vi "Main.vi"() -> ()   [LabVIEW 2017, in "CL_G3_BuilderApplicationLayer.lvlib"]
uses:
  CL_G3_BuilderApplicationLayer.lvlib
  TypeDefs/Organizational Types View.ctl
  TypeDefs/Email Behavior.ctl
  Message Queue/Message Cluster.ctl
  Build Analyzer/Build Analyzer.lvclass
  TypeDefs/Application Model Build States.ctl
  Exports/Exports/Export.lvclass
  <userlib>/_Cirrus Logic/LabVIEW SCC API/Source/Abstract SCC/Abstract SCC API.lvclass
  Components/Component.lvclass
  Build Analyzer/Build Analyzer.lvclass/Build Analyzer.ctl
  Exports/Exports/Export.lvclass/Export.ctl
  Components/Component.lvclass/Component.ctl
  Commit Behavior/Commit/Commit.lvclass
  Commit Behavior/Commit/Commit.lvclass/Commit.ctl
  Build Analyzer/Accessors/Read Component Product Name -_ Unique Name.vi
  Build Analyzer/Accessors/Read Product Name - Unique Name.vi
  Exports/Exports/Accessors/Read Product Name.vi
  Exports/Exports/Accessors/Read Built Version.vi
  Exports/Exports/Accessors/Read Owning Component's Product Name.vi
  Components/Accessors/Read Component Operations Errors.vi
  Exports/Exports/Accessors/Read Commit behavior.vi
  Exports/Exports/Accessors/Read Component Root path.vi
  Exports/Exports/Accessors/Write Export Operation Errors.vi
  Exports/Exports/Accessors/Read Component Export Dir.vi
  Exports/Exports/Accessors/Read Export Artifacts for SCC.vi
  Exports/Exports/Accessors/Read unique Name.vi
  Commit Behavior/Commit/Accessors/Read Commit Operation Errors.vi
  Message Queue/Enqueue Message (Single).vi
  Message Queue/Enqueue Message (Array).vi
  <vilib>/smtpClient/Set Message Text.vi
  <vilib>/LVH/i3 JSON/JSON Parsing/Get Object Parameter Files/Get Object Parameter - Object.vi
  <vilib>/LVH/i3 JSON/JSON Parsing/Get Object Parameter Files/Get Object Parameter - Numeric.vi
  <vilib>/LVH/i3 JSON/JSON Parsing/Get Object Parameter Files/Get Object Parameter - Array.vi
  <vilib>/LVH/i3 JSON/JSON Parsing/Get Array Value at Index Files/Get Array Value at Index - String.vi
  <vilib>/LVH/i3 JSON/JSON Parsing/Get Object Parameter Files/Get Object Parameter - String.vi
  <userlib>/_OpenG.lib/array/array.llb/Filter 1D Array (String)__ogtk.vi
  <vilib>/ErrorRing/Error Ring.xnode
  Message Queue/Message Queue.lvlib
  <vilib>/smtpClient/LabVIEWSMTPClient.lvlib
  CL_G3_VIComponentBuilder.lvlib
  <vilib>/Utility/config.llb/NI_LVConfig.lvlib
  <vilib>/LVH/i3 JSON/i3-json.lvlib
panel:
  in  "Sender's Email Address":string
  in  "Outgoing Mail Server":string
  in  "Email Behavior":T1
  in  "Email Address":string[](array[string])
  in  "Component \\ Export View":T2=enum."Component View"
  in  "Auto Submit Behavior":T3(ring)=enum."No Auto Submit"
  in  "Sync Action":enum16{"No Sync", "Sync", "Force Sync"}(ring)=enum."Force Sync"
  out "error out":errorcluster
  in  "Shutdown":bool
  in  "Back":bool
  in  "Status":string="Analysis Complete. Select componets to build"
  in  "Next Button":bool
  in  "Build Phase":T4(tab)
  in  "Select all":bool
  in  "Select None":bool
  in  "Components to build":u16[](array[ring]) items=["Component Builder", "Component Template NIPKG VIP", "Custom Install Step Launcher", "LabVIEW Atlassian API", "LabVIEW Auto Documentation", "LabVIEW Container", "LabVIEW SCC API", "NI Package Manager API", "NI Package Manager Build Spec Utils"]
  in  "Build Type":T5(ring)
  in  "Exports":i32(listbox)=-1
  in  "Abort":bool
  in  "Failed Builds":i32(listbox)=-2
  in  "Successful Builds":i32(listbox)=-2
  in  "Submission Status":i32(listbox)
  # "Email Options"
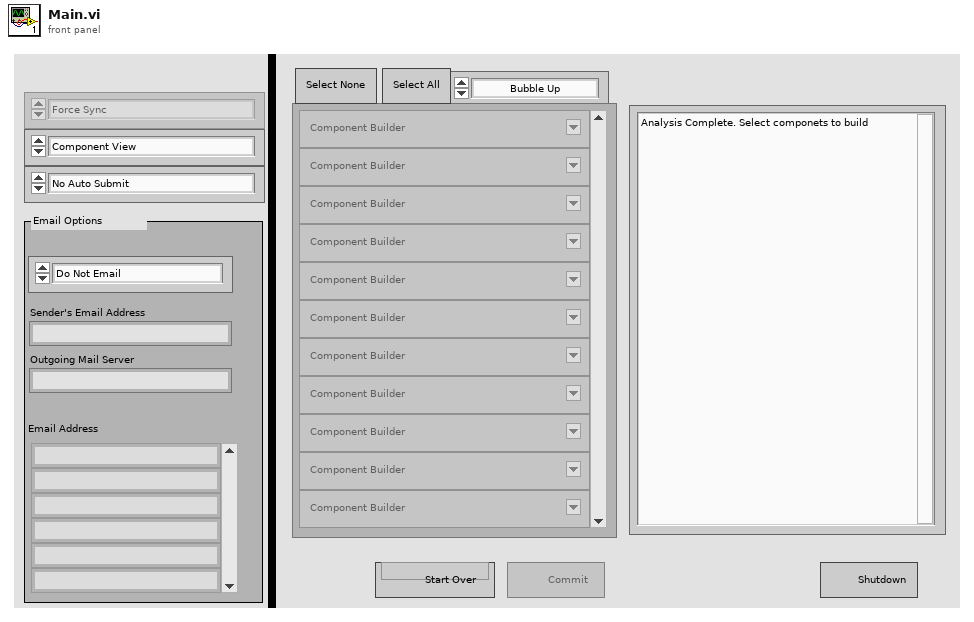
[diagram p1: front panel]
types:
  T1 = typedef "CL_G3_BuilderApplicationLayer.lvlib/Email Behavior.ctl" = enum16{"Do Not Email", "Email On Any Failure", "Email On All Successfully Built", "Email On Success OR Failure"}
  T2 = typedef "CL_G3_BuilderApplicationLayer.lvlib/Organizational Types View.ctl" = enum16{"Export View", "Component View"}
  T3 = enum16{"Auto Submit All Built Exports", "No Auto Submit"}
  T4 = enum32{"Configure Build", "Build Status", "Build Results", "Results"}
  T5 = enum16{"Bubble Up", "Build Dependencies", "Build Selected Only"}
  T6 = cluster{"This VI":refnum<vi>, "Build Analyzer":refnum<class "Build Analyzer.lvclass">, "Build Type":enum16{"Bubble Up", "Build Dependencies", "Build Selected Only"}, "Buildable Components":string[], "Components to Build":u16[], "Build Results":refnum<class "Export.lvclass">[], "Build Groups Folder":path, "View Type":T2, "Export Build Order":refnum<class "Export.lvclass">[], "Build Marker":u32, "Control References":cluster{"Auto Submit Behavior":refnum<vi>, "Email Address":refnum<vi>, "Outgoing Mail Server":refnum<vi>, "Sender's Email Address":refnum<vi>, "Sync Action":refnum<vi>, "Component \\ Export View Reference":refnum<vi>, "Email Behavior Reference":refnum<vi>, "Successful Builds":refnum<vi>, "Failed Builds":refnum<vi>, "Submission Status":refnum<vi>, "Shutdown":refnum<vi>, "Abort":refnum<vi>, "Front Panel":refnum<vi>, "Build Type":refnum<vi>, "Back":refnum<vi>, "Next":refnum<vi>, "Clear":refnum<vi>, "Select All":refnum<vi>, "Components to Build":refnum<vi>}}
  T7 = cluster{"SCC Session":refnum<class "Abstract SCC API.lvclass">, "Build Analyzer":refnum<class "Build Analyzer.lvclass">, "Ordered Exports":refnum<class "Export.lvclass">[], "Build Marker":u32, "Build Groups Folder":path, "Components":refnum<class "Component.lvclass">[], "Sync Action":enum16{"No Sync", "Sync", "Force Sync"}, "Build Options i3JSON Tree":variant, "Broadcast Server Id":refnum<k5>, "Failed Submissions":refnum<class "Export.lvclass">[], "All Attempted Submissions":refnum<class "Export.lvclass">[], "Successful Submissions":refnum<class "Export.lvclass">[], "SCC Synchronized Paths":variant, "Snapshot Depot Directories":string[]}
  T8 = typedef "CL_G3_BuilderApplicationLayer.lvlib/Application Model Build States.ctl" = enum32{"Configure Build", "Build Pre Check", "Build Status", "Build Results", "Finished"}
  T9 = cluster{"Dynamic Event":refnum<user-event>, "Build Analyzer":refnum<class "Build Analyzer.lvclass">, "Current Phase":T8, "Email Behavior":T1, "Export Build Order":refnum<class "Export.lvclass">[]}
  T10 = typedef "CL_G3_BuilderApplicationLayer.lvlib/Message Queue.lvlib/Message Cluster.ctl" = cluster{"Message":string, "Message Data":variant}
  T11 = typedef "CL_G3_BuilderApplicationLayer.lvlib/Message Queue.lvlib/All Message Queues.ctl" = cluster{"UI":refnum<queue>, "Application Model":refnum<queue>, "UI manager":refnum<queue>, "Build Engine":refnum<queue>}
  T12 = enum8{"Enabled", "Disabled", "Disabled and Grayed Out"}
  T13 = cluster{"Ordered Exports":refnum<class "Export.lvclass">[], "Build Groups Folder":path}
  T14 = typedef "LabVIEWSMTPClient.lvlib/SmtpClientHandle.ctl" = refnum<k1>
  T15 = cluster{"Ordered Exports":refnum<class "Export.lvclass">[], "Build Marker":u32, "Build Groups Folder":path, "Build Engine Queue":refnum<queue>, "error out":errorcluster}
  T16 = cluster{"Export Path":path, "Export Files":string[]}
  T17 = typedef "NI_LVConfig.lvlib/Config Data RefNum.ctl" = refnum<k1>
  T18 = cluster{"SCC Session":refnum<class "Abstract SCC API.lvclass">, "Failed Submissions":refnum<class "Export.lvclass">[], "All Exports":refnum<class "Export.lvclass">[], "Exports W\\O Errors":refnum<class "Export.lvclass">[], "Ordered Expors":refnum<class "Export.lvclass">[]}
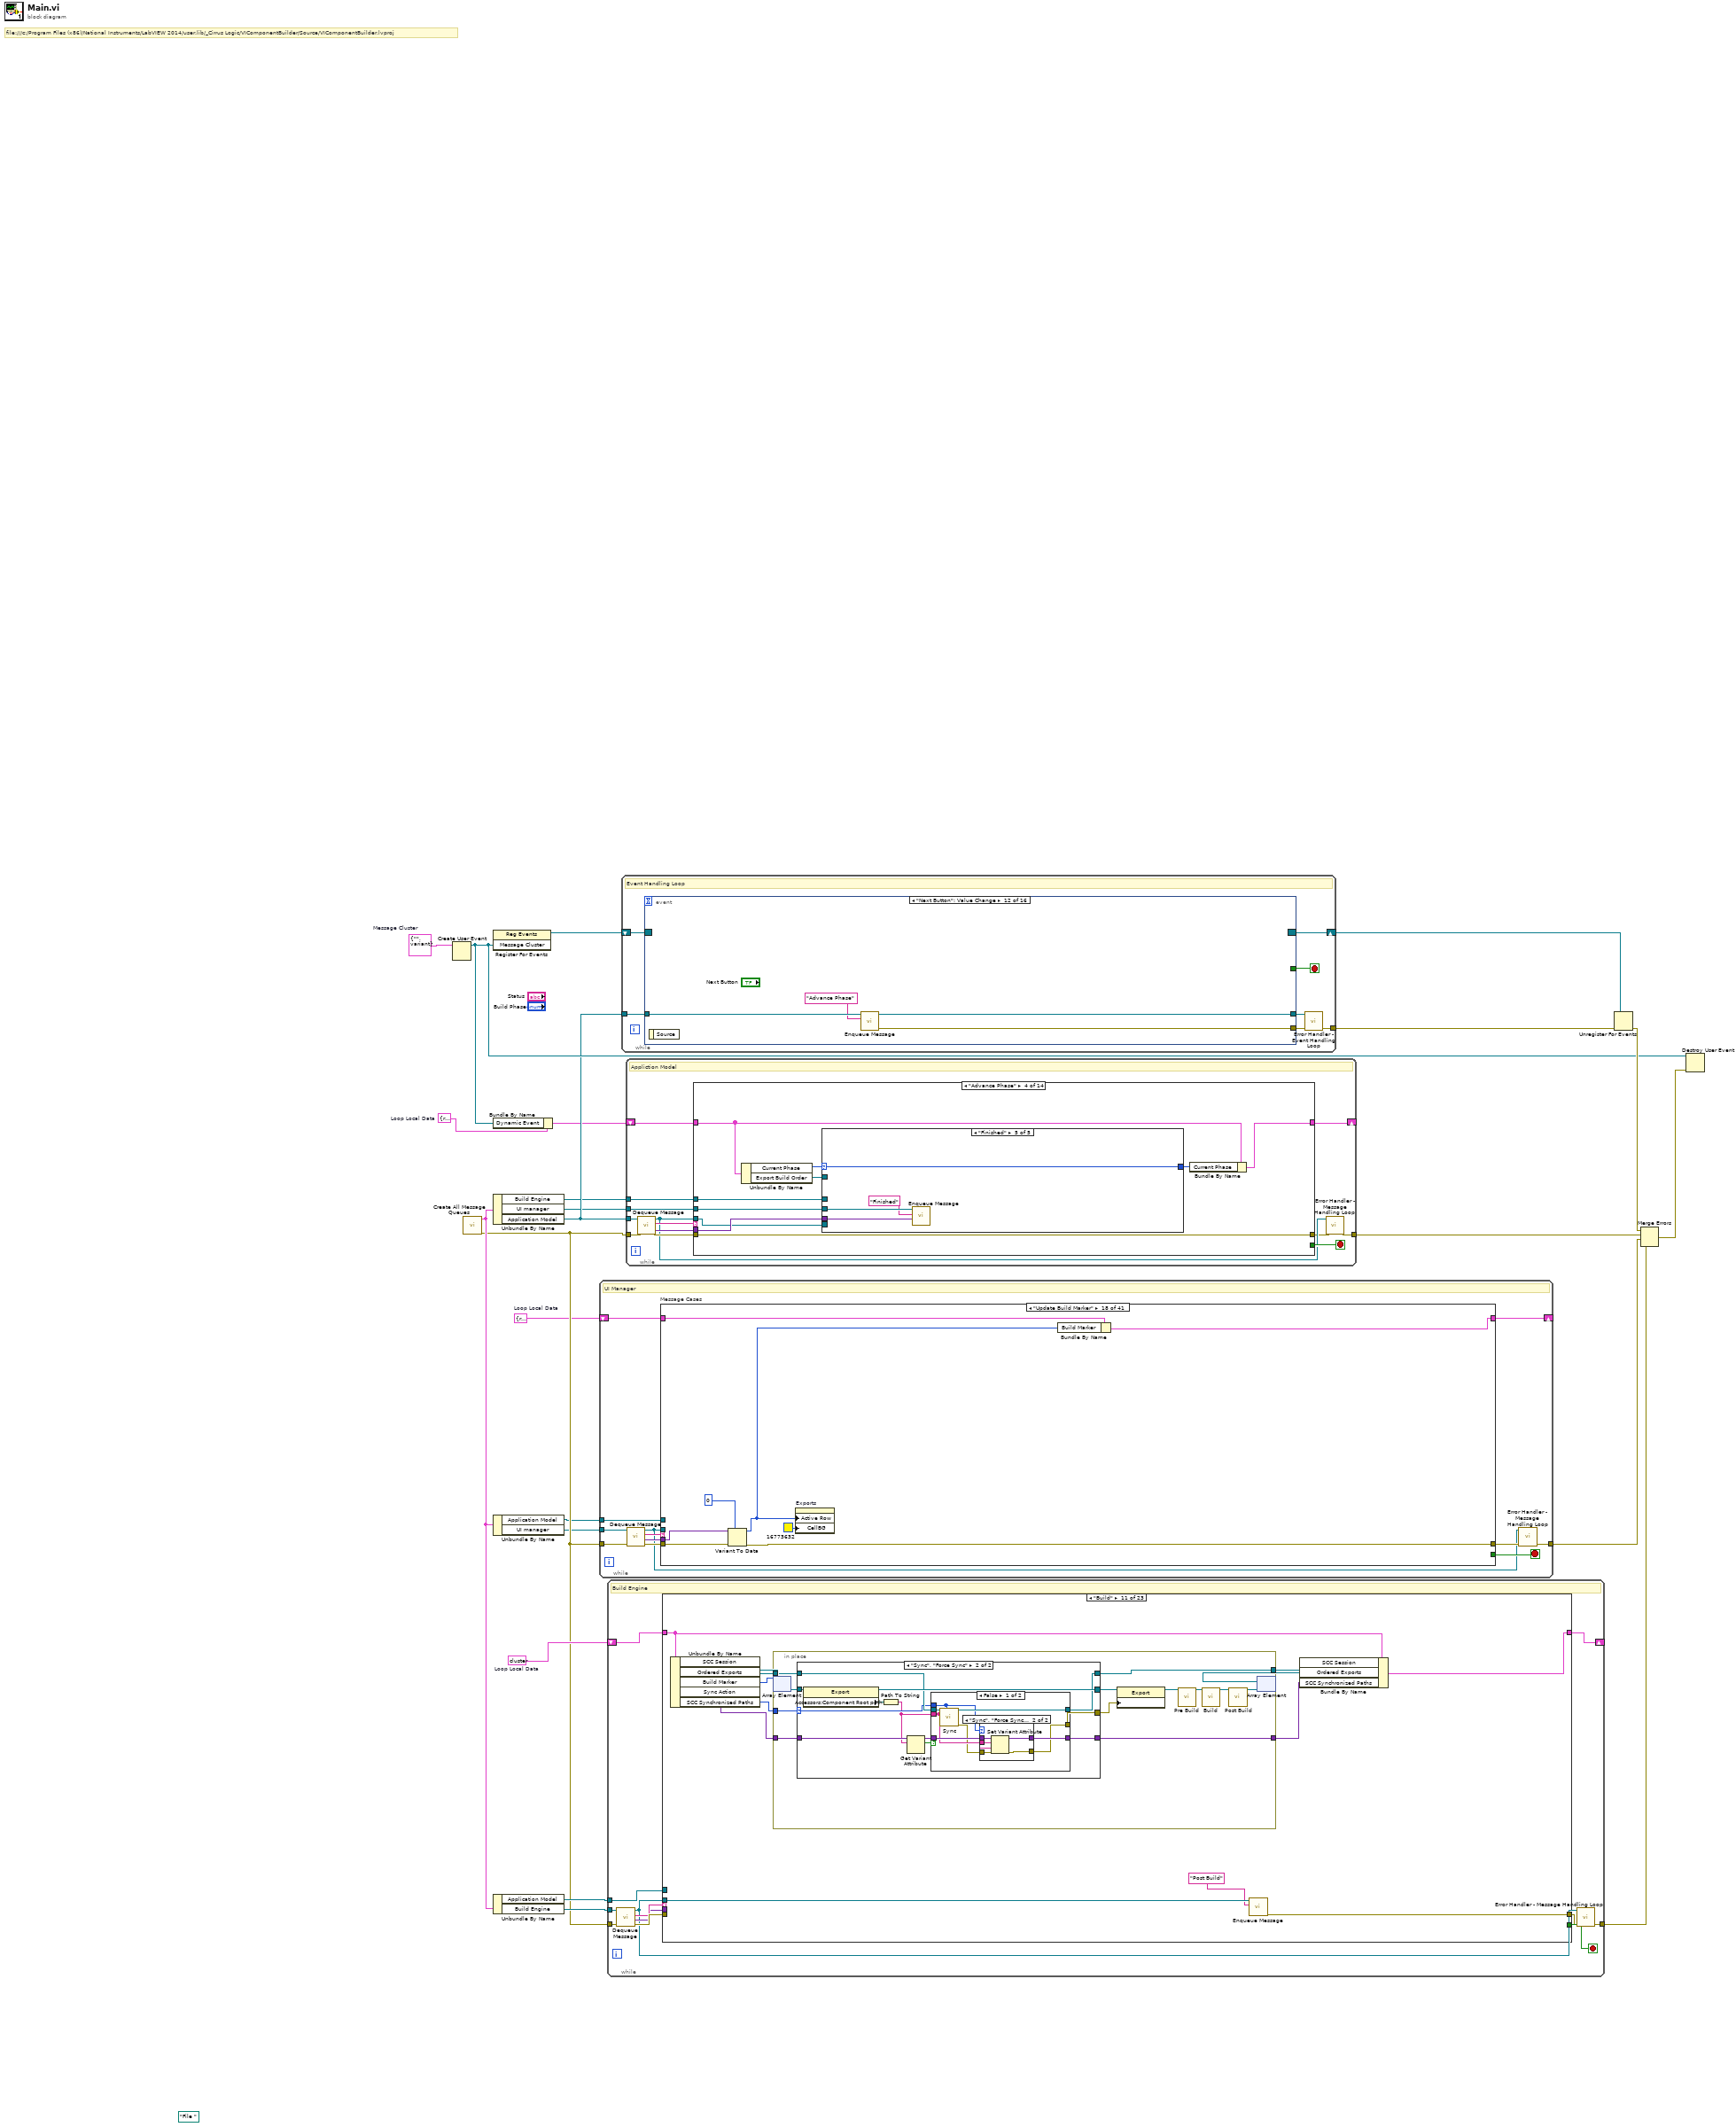
[diagram p0: block diagram]
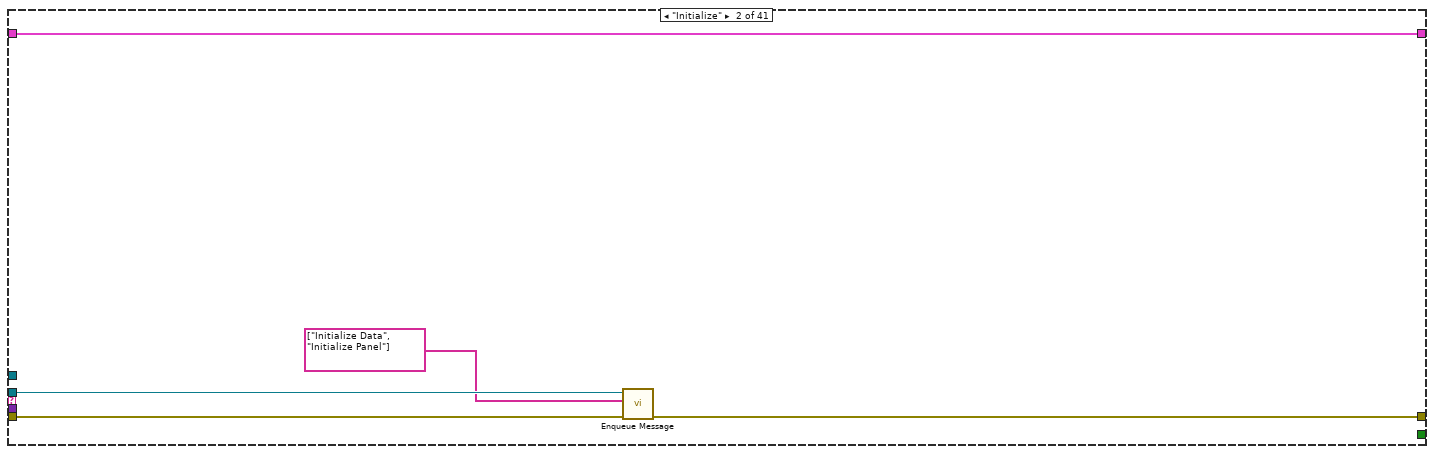
[diagram p3: hidden frame]
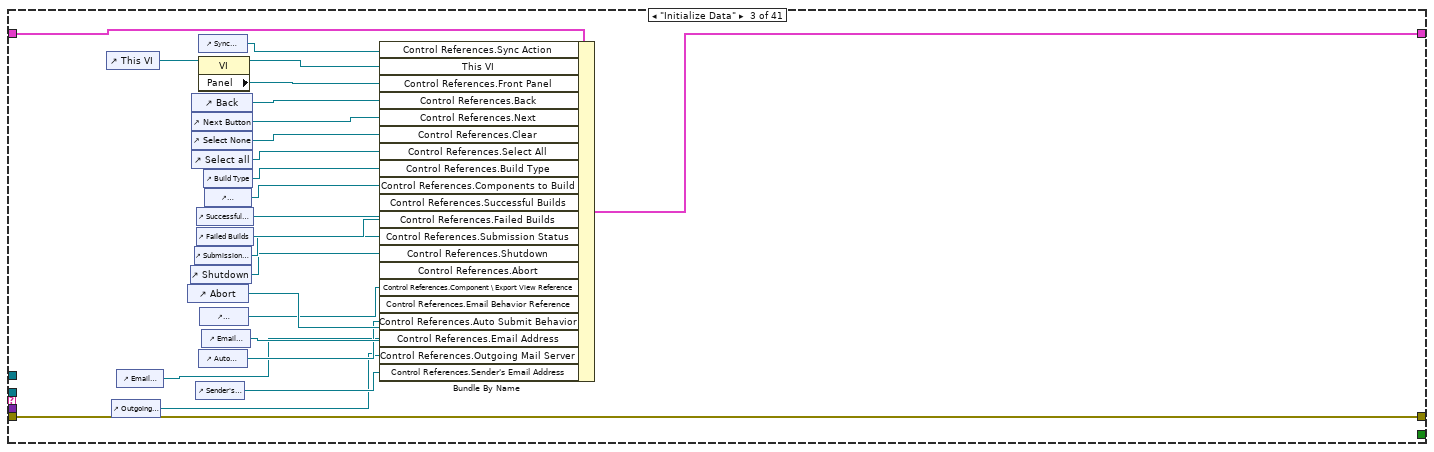
[diagram p4: hidden frame]
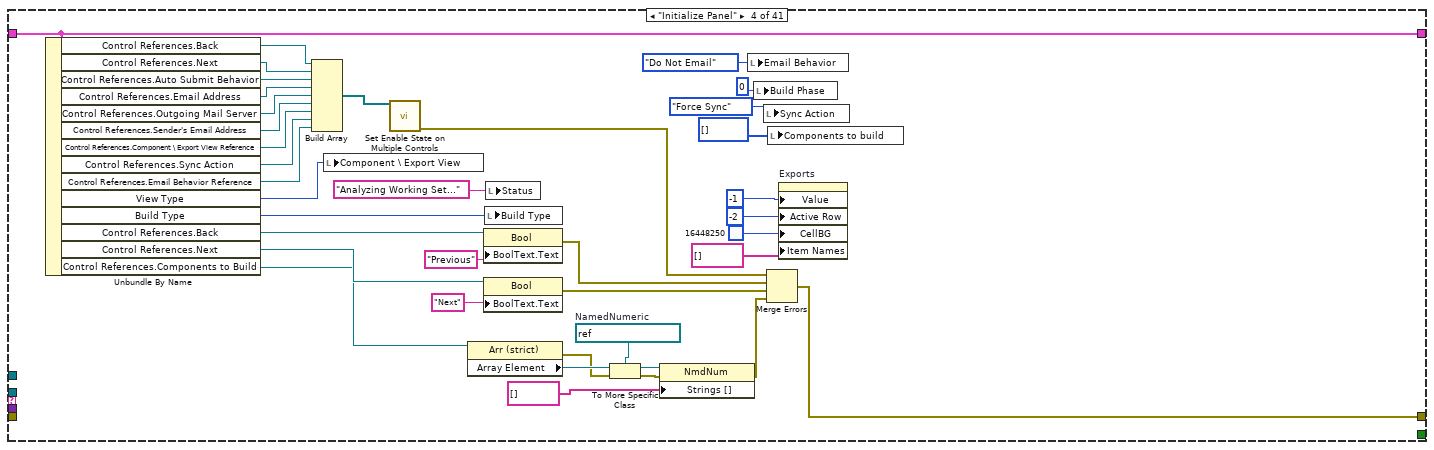
[diagram p5: hidden frame]
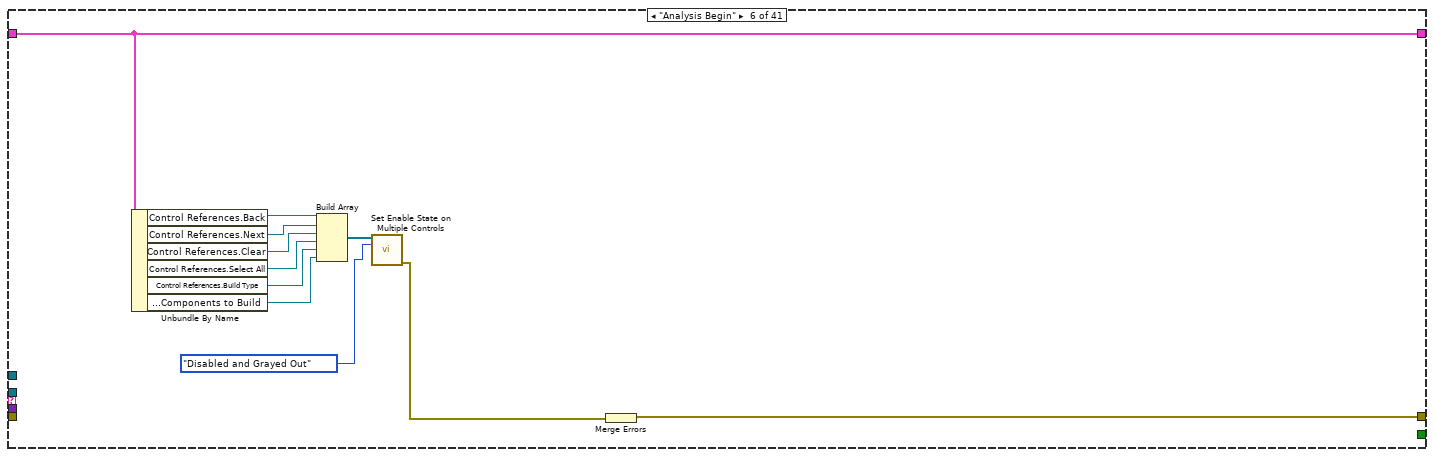
[diagram p7: hidden frame]
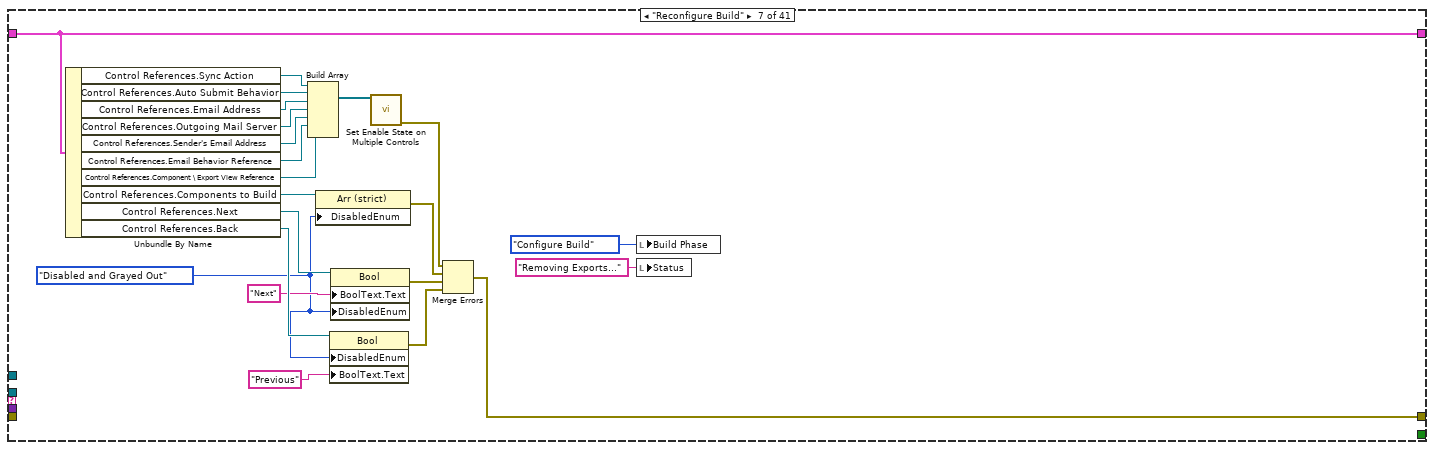
[diagram p8: hidden frame]
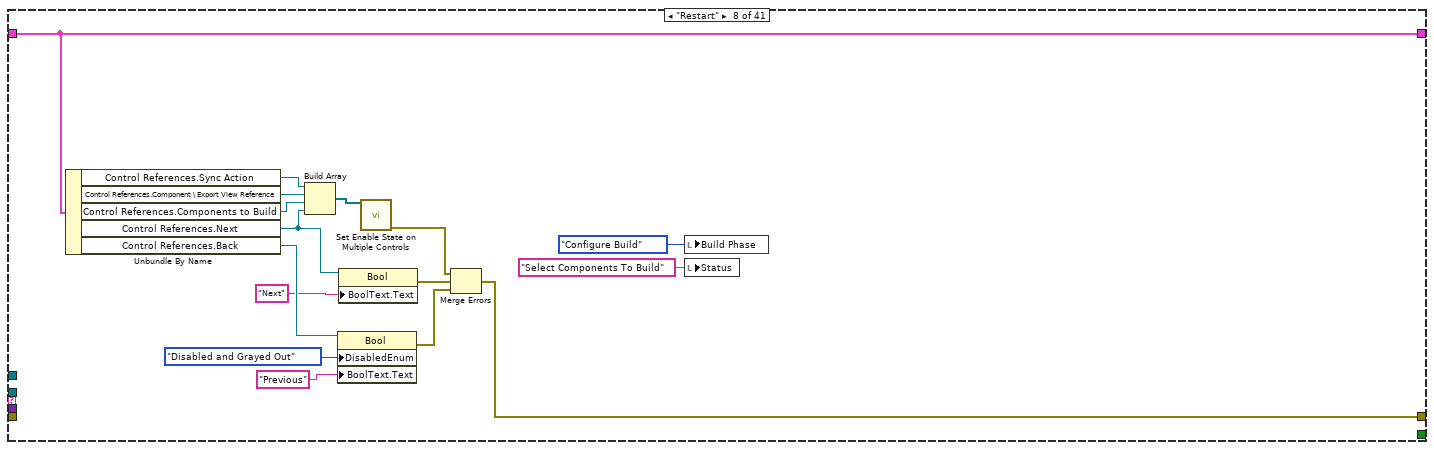
[diagram p9: hidden frame]
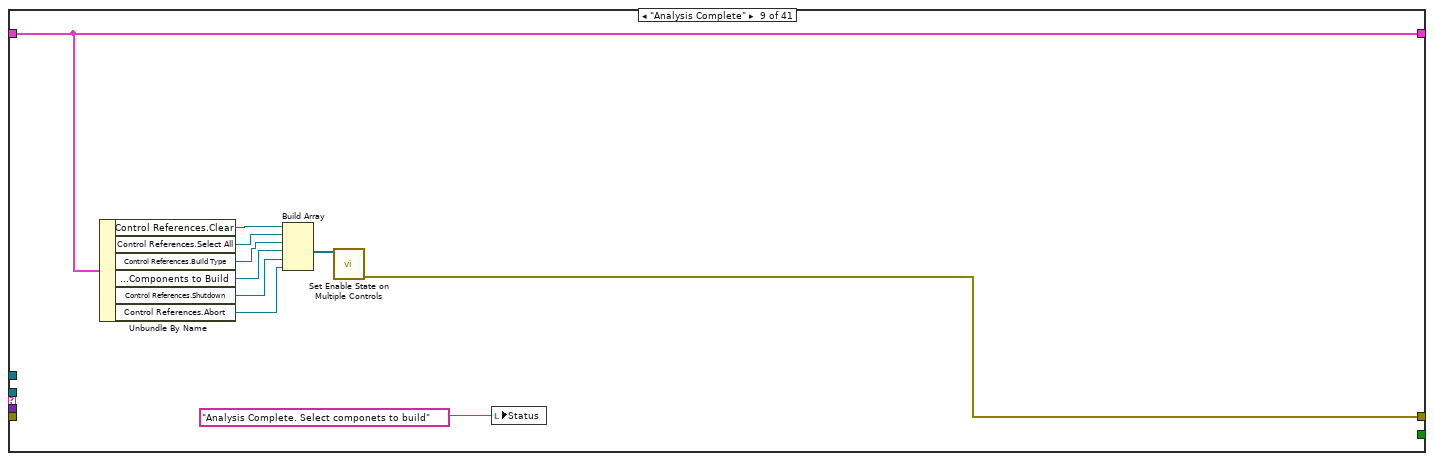
[diagram p10: hidden frame]
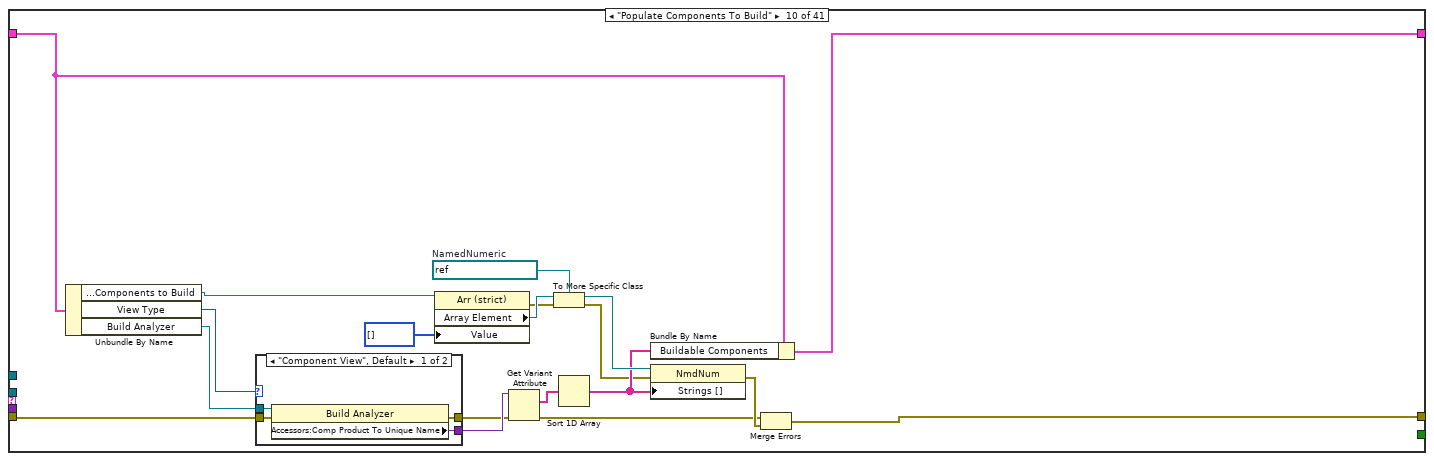
[diagram p11: hidden frame]
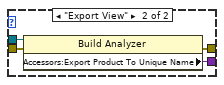
[diagram p12: hidden frame]
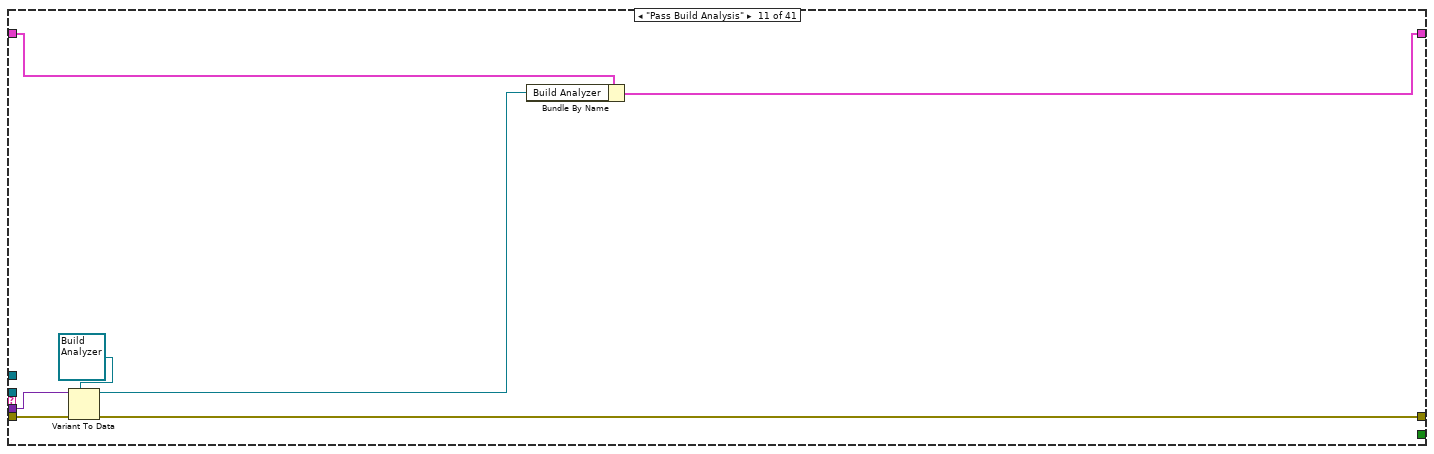
[diagram p13: hidden frame]
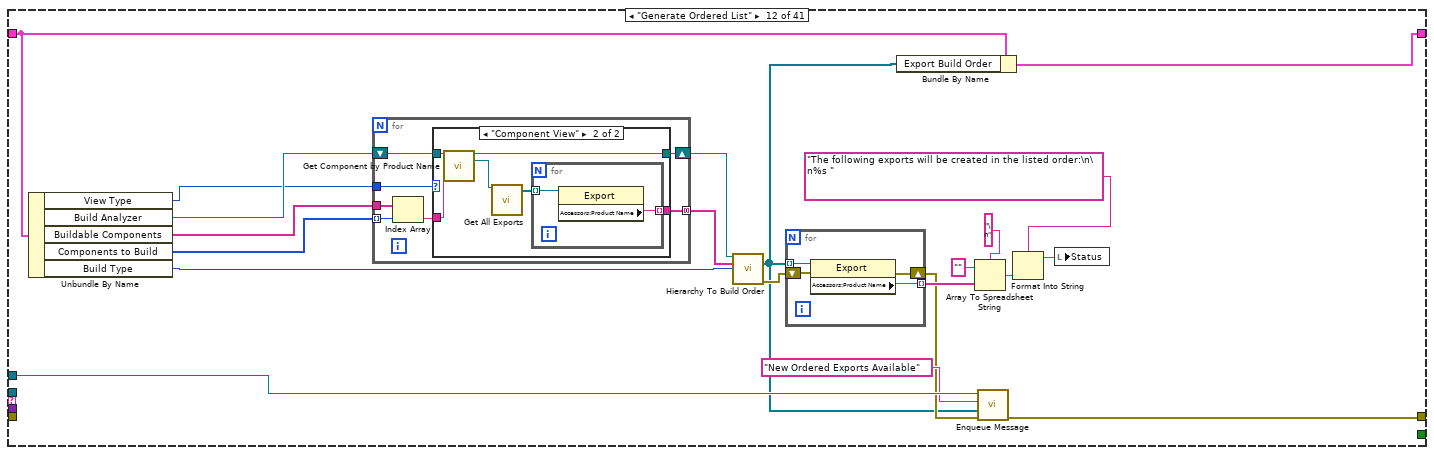
[diagram p14: hidden frame]
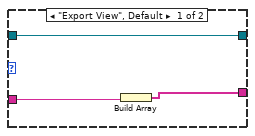
[diagram p15: hidden frame]
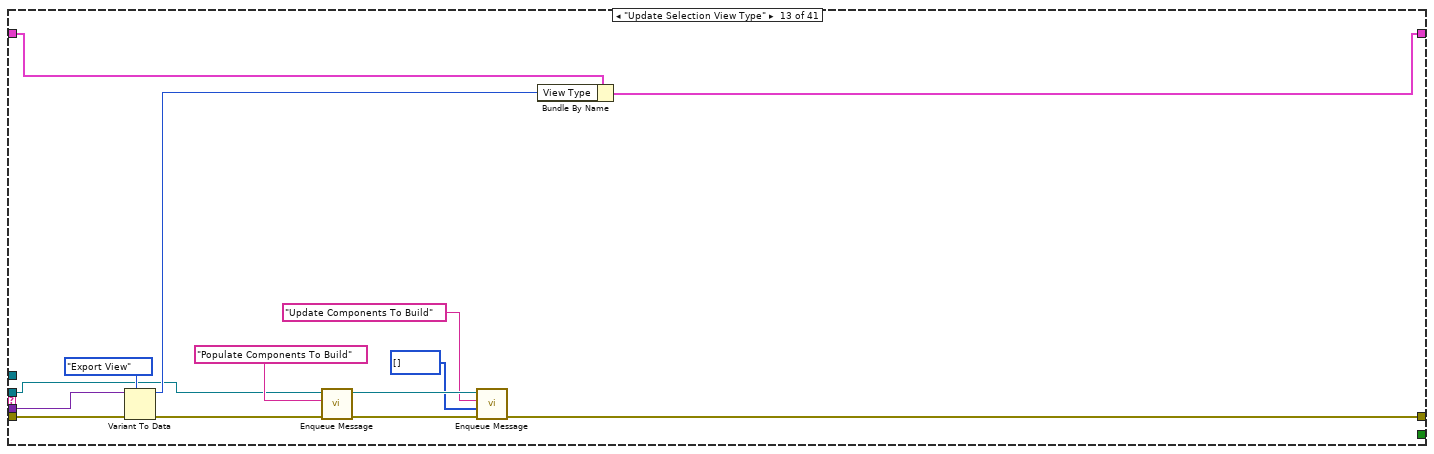
[diagram p16: hidden frame]
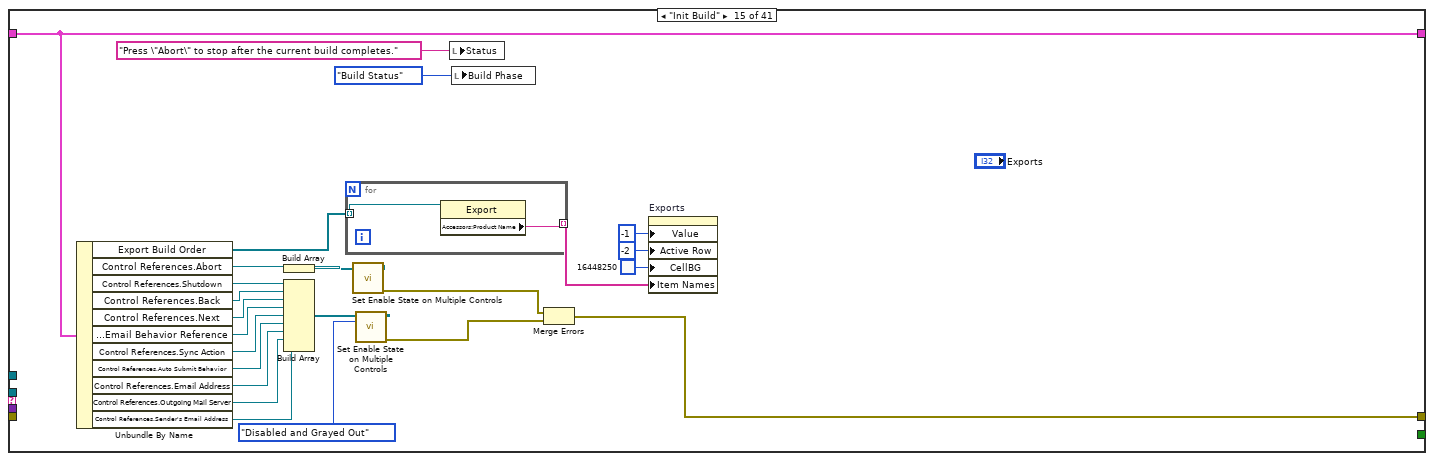
[diagram p18: hidden frame]
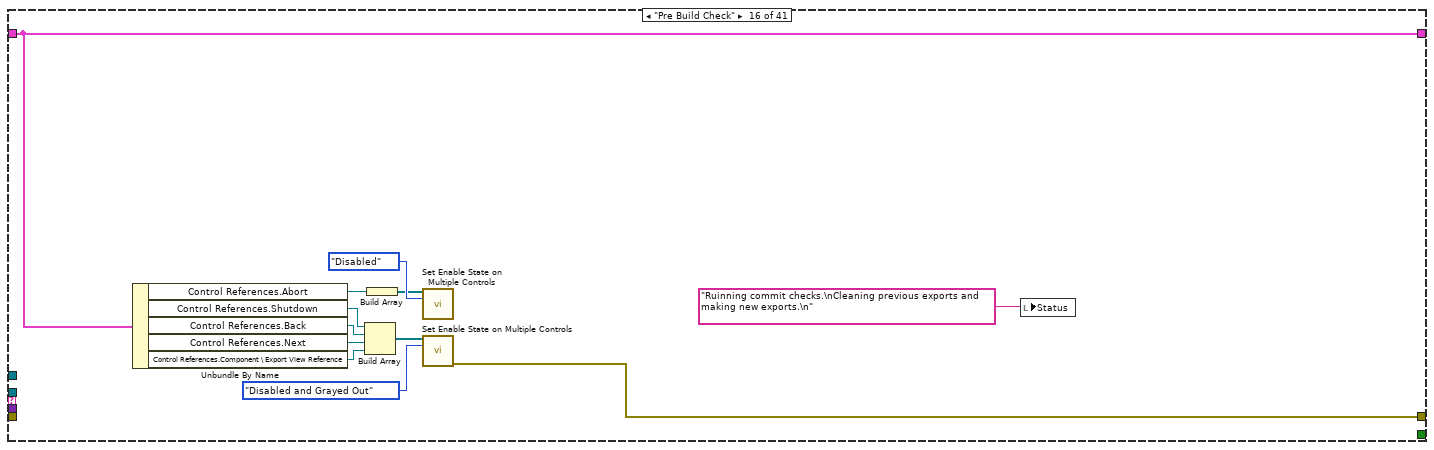
[diagram p19: hidden frame]
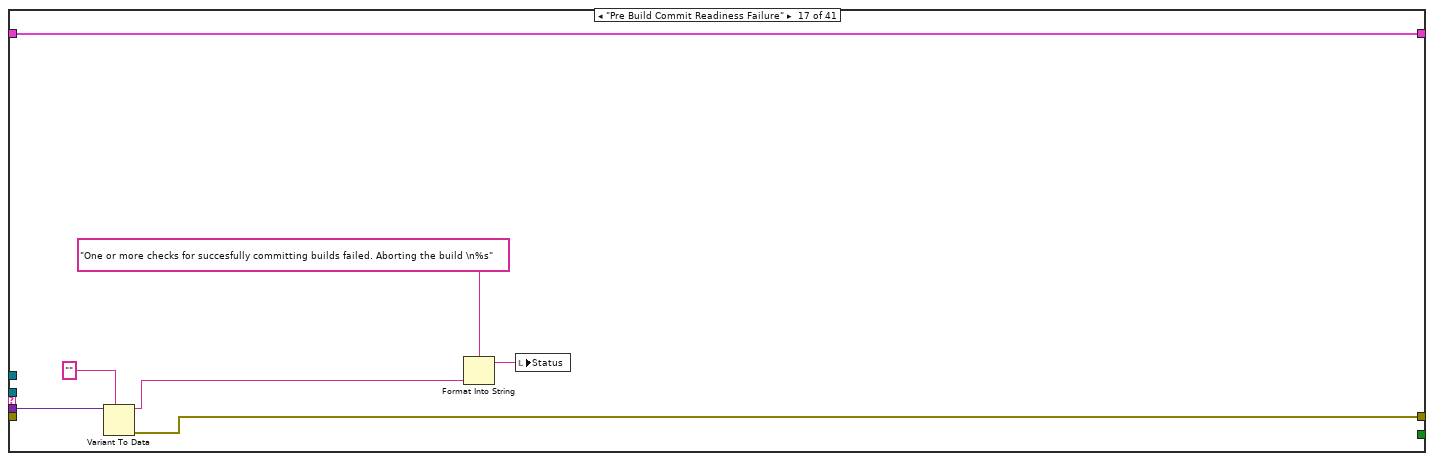
[diagram p20: hidden frame]
diagram:
  w3 = T6 {"This VI"=refnum, "Build Analyzer"=refnum, "Build Type"=enum."Bubble Up", "Buildable Components"=[], "Components to Build"=[], "Build Results"=[], "Build Groups Folder"=path "", "View Type"=enum."Component View", "Export Build Order"=[], "Build Marker"=0, "Control References"={"Auto Submit Behavior"=refnum, "Email Address"=refnum, "Outgoing Mail Server"=refnum, "Sender's Email Address"=refnum, "Sync Action"=refnum, "Component \\ Export View Reference"=refnum, "Email Behavior Reference"=refnum, "Successful Builds"=refnum, "Failed Builds"=refnum, "Submission Status"=refnum, "Shutdown"=refnum, "Abort"=refnum, "Front Panel"=refnum, "Build Type"=refnum, "Back"=refnum, "Next"=refnum, "Clear"=refnum, "Select All"=refnum, "Components to Build"=refnum}}  # Loop Local Data
  (unwired) path "File "
  w15 = T7 {"SCC Session"=refnum, "Build Analyzer"=refnum, "Ordered Exports"=[], "Build Marker"=0, "Build Groups Folder"=path "", "Components"=[], "Sync Action"=enum."Force Sync", "Build Options i3JSON Tree"=variant, "Broadcast Server Id"=refnum, "Failed Submissions"=[], "All Attempted Submissions"=[], "Successful Submissions"=[], "SCC Synchronized Paths"=variant, "Snapshot Depot Directories"=[]}  # Loop Local Data
  w20 = T9 {"Dynamic Event"=refnum, "Build Analyzer"=refnum, "Current Phase"=enum."Configure Build", "Email Behavior"=enum."Do Not Email", "Export Build Order"=[]}  # Loop Local Data
  w21 = T10 {"Message"="", "Message Data"=variant}  # Message Cluster
  # "file:///c:/Program Files (x86)/National Instruments/LabVIEW 2014/user.lib/_Cirrus Logic/VIComponentBuilder/Source/VIComponentBuilder.lvproj"
  n1 = Create User Event(user event datatype=w21) -> (user event=w13:refnum<user-event>)  [unwired: 1 in, 1 out]
  n2 = call "Create All Message Queues.vi"() -> ("error out"=w11:errorcluster, "Message Queues out"=w12:T11)  [unwired: 10 in]
  n3 = register-events(w13) -> (reference out=w7:refnum<event-registration>)  [unwired: 2 in, 1 out]
  n4 = Bundle By Name(cluster=w20, "Dynamic Event"=w13) -> (w1:T9)
  n5 = Unbundle By Name(w12) -> ("Build Engine"=w6:refnum<queue>, "UI manager"=w5:refnum<queue>, "Application Model"=w10:refnum<queue>)
  n6 = Unbundle By Name(w12) -> ("Application Model"=w2:refnum<queue>, "UI manager"=w4:refnum<queue>)
  n7 = Unbundle By Name(w12) -> ("Application Model"=w14:refnum<queue>, "Build Engine"=w19:refnum<queue>)
  n8 = while {
    tunnel: w4 -> [w28]
    shift-right: [w34] -> _
    shift-left: w3 -> [w35]
    tunnel: w11 -> [w32]
    tunnel: [w25] -> w18
    tunnel: w2 -> [w27]
    stop <- w33 stop-if-true
    # "UI Manager"
    n9 = call "Dequeue Message.vi"("error in (no error)"=w32, "Message Queue"=w28) -> ("error out"=w31:errorcluster, "Message Data"=w29:variant, "Message"=w30:string, "dup Message Queue"=w24:refnum<queue>)  [unwired: 6 in]
    n10 = case "Message Cases" shown="\"Update Build Marker\"" w30 {
      selector: w30 -> [_ _ _ _ _ _ _ _ _ _ _ _ _ _ _ _ _ _ _ _ _ _ _ _ _ _ _ _ _ _ _ _ _ _ _ _ _ w691 _ _ _]
      tunnel: w24 -> [_ w40 _ _ _ _ _ _ _ _ _ _ w248 _ _ _ _ _ _ _ _ _ _ _ _ w536 _ _ _ _ _ _ _ _ _ w678 _ _ _ _ w712]
      tunnel: w31 -> [w37 w41 w55 _ w106 _ _ _ _ w167 w196 _ w253 w258 _ _ _ w308 w312 w345 _ w451 _ _ _ _ _ _ w572 _ _ _ w610 w629 _ w673 w690 _ w702 _ _]
      tunnel: [w37 w42 w55 w87 w106 w111 w131 w148 w160 w173 w195 w210 w245 w258 w264 w287 w301 w307 w313 w322 w359 w451 w452 w468 w519 w530 w548 w563 w572 w574 w584 w593 w610 w628 w648 w674 w683 w692 w702 w703 w709] -> w26
      tunnel: w35 -> [w36 w38 w66 w103 w105 w117 w139 w155 w165 w176 w199 w220 w256 w257 w282 w296 w303 w311 w318 w350 w364 w450 w456 w467 w522 w535 w547 w562 w571 w579 w586 w591 w611 w631 w656 w677 w689 w693 w701 w706 w715]
      tunnel: [w36 w38 w65 w103 w105 w117 w139 w155 w165 w177 w194 w201 w255 w257 w282 w296 w303 w305 w318 w349 w364 w450 w456 w466 w524 w537 w547 w562 w571 w579 w586 w591 w613 w633 w654 w677 w689 w693 w701 w705 w714] -> w34
      tunnel: [_ _ _ _ _ _ _ _ _ _ _ _ _ _ _ _ _ _ _ _ _ _ _ _ _ _ _ _ _ _ _ _ _ _ _ TRUE _ _ _ _ _] -> w33
      tunnel: w29 -> [_ _ _ _ _ _ _ _ _ _ w197 _ w254 _ _ _ w302 w309 w316 w346 w362 _ _ _ _ w538 w550 w565 _ _ w585 w595 _ w630 w660 _ w688 _ _ w707 w717]
      tunnel: w27 -> [_ _ _ _ _ _ _ _ _ _ _ w212 _ _ _ _ _ _ _ _ _ _ _ w475 _ _ _ _ _ _ _ _ _ _ _ _ w680 _ _ _ _]
      frame "---Initialize---" {
      }
      frame "Initialize" {
        # "Initialize - Send separate messages to initialize the data and the front panel.  Bundle control references."
        n11 = call-poly "Enqueue Message.vi"("error in (no error)"=w41, "Message Array"=string[] ["Initialize Data", "Initialize Panel"], "Message Queue"=w40) -> ("error out"=w42:errorcluster)  [unwired: 7 in, 1 out]
      }
      frame "Initialize Data" {
        # "Initialize Data - Initialize the state data cluster."
        n12 = control-ref of="This VI"() -> (w52:refnum<vi>)
        n13 = control-ref of="Outgoing Mail Server"() -> (w43:refnum<vi>)
        n14 = control-ref of="Email Address"() -> (w44:refnum<vi>)
        n15 = control-ref of="Abort"() -> (w53:refnum<vi>)
        n16 = control-ref of="Shutdown"() -> (w54:refnum<vi>)
        n17 = control-ref of="Back"() -> (w64:refnum<vi>)
        n18 = control-ref of="Next Button"() -> (w63:refnum<vi>)
        n19 = control-ref of="Select None"() -> (w62:refnum<vi>)
        n20 = control-ref of="Select all"() -> (w61:refnum<vi>)
        n21 = control-ref of="Submission Status"() -> (w56:refnum<vi>)
        n22 = control-ref of="Sender's Email Address"() -> (w45:refnum<vi>)
        n23 = control-ref of="Successful Builds"() -> (w58:refnum<vi>)
        n24 = control-ref of="Failed Builds"() -> (w57:refnum<vi>)
        n25 = control-ref of="Sync Action"() -> (w47:refnum<vi>)
        n26 = property class="VI"(reference=w52) -> (reference out=w51:refnum<vi>, "Panel"=w50:refnum<vi>)  [unwired: 1 in, 1 out]
        n27 = control-ref of="Auto Submit Behavior"() -> (w46:refnum<vi>)
        n28 = control-ref of="Component \\ Export View"() -> (w49:refnum<vi>)
        n29 = control-ref of="Email Behavior"() -> (w48:refnum<vi>)
        n30 = control-ref of="Build Type"() -> (w60:refnum<vi>)
        n31 = control-ref of="Components to build"() -> (w59:refnum<vi>)
        n32 = Bundle By Name(cluster=w66, "Control References.Sync Action"=w47, "This VI"=w51, "Control References.Front Panel"=w50, "Control References.Back"=w64, "Control References.Next"=w63, "Control References.Clear"=w62, "Control References.Select All"=w61, "Control References.Build Type"=w60, "Control References.Components to Build"=w59, "Control References.Successful Builds"=w58, "Control References.Failed Builds"=w57, "Control References.Submission Status"=w56, "Control References.Shutdown"=w54, "Control References.Abort"=w53, "Control References.Component \\ Export View Reference"=w49, "Control References.Email Behavior Reference"=w48, "Control References.Auto Submit Behavior"=w46, "Control References.Email Address"=w44, "Control References.Outgoing Mail Server"=w43, "Control References.Sender's Email Address"=w45) -> (w65:T6)
      }
      frame "Initialize Panel" {
        w94 = refnum<vi> refnum  # NamedNumeric
        # "Initialize Panel - Initialize the appearance of the front panel here."
        n33 = Unbundle By Name(w103) -> ("Control References.Back"=w69:refnum<vi>, "Control References.Next"=w68:refnum<vi>, "Control References.Auto Submit Behavior"=w70:refnum<vi>, "Control References.Email Address"=w71:refnum<vi>, "Control References.Outgoing Mail Server"=w72:refnum<vi>, "Control References.Sender's Email Address"=w73:refnum<vi>, "Control References.Component \\ Export View Reference"=w78:refnum<vi>, "Control References.Sync Action"=w77:refnum<vi>, "Control References.Email Behavior Reference"=w76:refnum<vi>, "View Type"=w84:T2, "Build Type"=w85:T5, "Control References.Back"=w102:refnum<vi>, "Control References.Next"=w101:refnum<vi>, "Control References.Components to Build"=w95:refnum<vi>)
        n34 = Build Array(w69, w68, w70, w71, w72, w73, w78, w77, w76) -> (w75:refnum<vi>[])
        n35 = local write "Component \\ Export View"(w84) -> ()
        n36 = call "Set Enable State on Multiple Controls.vi"("Control References"=w75) -> ("error out"=w74:errorcluster)  [unwired: 13 in, 1 out]
        n37 = property class="Arr (strict)"(reference=w95) -> (error out=w89:errorcluster, "Array Element"=w91:refnum<vi>)  [unwired: 1 in, 1 out]
        n38 = property class="Bool"(reference=w102, "BoolText.Text"="Previous" ("Boolean Text.Text")) -> (error out=w98:errorcluster)  [unwired: 1 in, 1 out]
        n39 = property class="Bool"(reference=w101, "BoolText.Text"="Next" ("Boolean Text.Text")) -> (error out=w97:errorcluster)  [unwired: 1 in, 1 out]
        n40 = local write "Build Type"(w85) -> ()
        n41 = local write "Status"("Analyzing Working Set..." ("Status")) -> ()
        n42 = To More Specific Class(target class=w94, reference=w91, error in=w89) -> (specific class reference=w93:refnum<vi>, error out=w92:errorcluster)
        n43 = property on="Property Node" class="NmdNum"(reference=w93, error in=w92, "Strings []"=string[] []) -> (error out=w88:errorcluster)  [unwired: 1 out]
        n44 = local write "Email Behavior"(Email_Behavior."Do Not Email" ("Email Behavior")) -> ()
        n45 = local write "Build Phase"(0) -> ()
        n46 = local write "Sync Action"(enum16{"No Sync", "Sync", "Force Sync"}."Force Sync" ("Sync Action")) -> ()
        n47 = Merge Errors(w74, w98, w97, w88) -> (w87:errorcluster)
        n48 = local write "Components to build"(i32[] [] ("Components to build")) -> ()
        n49 = property on="Exports" class="LstBox (strict)"("Value"=-1 ("Exports"), "Active Row"=-2 ("Active Row:Active Row Number"), "CellBG"=u32 16448250, "Item Names"=string[] []) -> ()  [unwired: 2 in, 2 out]
      }
      frame "---Analyze---" {
      }
      frame "Analysis Begin" {
        n50 = Unbundle By Name(w117) -> ("Control References.Back"=w116:refnum<vi>, "Control References.Next"=w115:refnum<vi>, "Control References.Clear"=w114:refnum<vi>, "Control References.Select All"=w113:refnum<vi>, "Control References.Build Type"=w112:refnum<vi>, "Control References.Components to Build"=w110:refnum<vi>)
        n51 = Build Array(w116, w115, w114, w113, w112, w110) -> (w109:refnum<vi>[])
        n52 = call "Set Enable State on Multiple Controls.vi"("Control References"=w109, "State"=T12."Disabled and Grayed Out" ("Disabled")) -> ("error out"=w107:errorcluster)  [unwired: 12 in, 1 out]
        n53 = Merge Errors(w107) -> (w111:errorcluster)
      }
      frame "Reconfigure Build" {
        w129 = T12."Disabled and Grayed Out" ("Disabled")
        n54 = Unbundle By Name(w139) -> ("Control References.Sync Action"=w118:refnum<vi>, "Control References.Auto Submit Behavior"=w126:refnum<vi>, "Control References.Email Address"=w125:refnum<vi>, "Control References.Outgoing Mail Server"=w124:refnum<vi>, "Control References.Sender's Email Address"=w123:refnum<vi>, "Control References.Email Behavior Reference"=w122:refnum<vi>, "Control References.Component \\ Export View Reference"=w121:refnum<vi>, "Control References.Components to Build"=w130:refnum<vi>, "Control References.Next"=w136:refnum<vi>, "Control References.Back"=w138:refnum<vi>)
        n55 = Build Array(w118, w126, w125, w124, w123, w122, w121) -> (w120:refnum<vi>[])
        n56 = property class="Arr (strict)"(reference=w130, "DisabledEnum"=w129) -> (error out=w128:errorcluster)  [unwired: 1 in, 1 out]
        n57 = property class="Bool"(reference=w138, "DisabledEnum"=w129, "BoolText.Text"="Previous" ("Boolean Text.Text")) -> (error out=w132:errorcluster)  [unwired: 1 in, 1 out]
        n58 = property class="Bool"(reference=w136, "BoolText.Text"="Next" ("Boolean Text.Text"), "DisabledEnum"=w129) -> (error out=w133:errorcluster)  [unwired: 1 in, 1 out]
        n59 = call "Set Enable State on Multiple Controls.vi"("Control References"=w120) -> ("error out"=w119:errorcluster)  [unwired: 13 in, 1 out]
        n60 = Merge Errors(w119, w128, w133, w132) -> (w131:errorcluster)
        n61 = local write "Build Phase"(T4."Configure Build" ("Build Phase")) -> ()
        n62 = local write "Status"("Removing Exports..." ("Status")) -> ()
      }
      frame "Restart" {
        n63 = Unbundle By Name(w155) -> ("Control References.Sync Action"=w140:refnum<vi>, "Control References.Component \\ Export View Reference"=w145:refnum<vi>, "Control References.Components to Build"=w144:refnum<vi>, "Control References.Next"=w141:refnum<vi>, "Control References.Back"=w154:refnum<vi>)
        n64 = Build Array(w140, w145, w144, w141) -> (w143:refnum<vi>[])
        n65 = property class="Bool"(reference=w154, "DisabledEnum"=T12."Disabled and Grayed Out" ("Disabled"), "BoolText.Text"="Previous" ("Boolean Text.Text")) -> (error out=w149:errorcluster)  [unwired: 1 in, 1 out]
        n66 = property class="Bool"(reference=w141, "BoolText.Text"="Next" ("Boolean Text.Text")) -> (error out=w150:errorcluster)  [unwired: 1 in, 1 out]
        n67 = call "Set Enable State on Multiple Controls.vi"("Control References"=w143) -> ("error out"=w142:errorcluster)  [unwired: 13 in, 1 out]
        n68 = Merge Errors(w142, w150, w149) -> (w148:errorcluster)
        n69 = local write "Build Phase"(T4."Configure Build" ("Build Phase")) -> ()
        n70 = local write "Status"("Select Components To Build" ("Status")) -> ()
      }
      frame "Analysis Complete" {
        n71 = Unbundle By Name(w165) -> ("Control References.Clear"=w164:refnum<vi>, "Control References.Select All"=w163:refnum<vi>, "Control References.Build Type"=w162:refnum<vi>, "Control References.Components to Build"=w159:refnum<vi>, "Control References.Shutdown"=w158:refnum<vi>, "Control References.Abort"=w157:refnum<vi>)
        n72 = Build Array(w164, w163, w162, w159, w158, w157) -> (w156:refnum<vi>[])
        n73 = call "Set Enable State on Multiple Controls.vi"("Control References"=w156) -> ("error out"=w160:errorcluster)  [unwired: 13 in, 1 out]
        n74 = local write "Status"("Analysis Complete. Select componets to build" ("Status")) -> ()
      }
      frame "Populate Components To Build" {
        w184 = refnum<vi> refnum  # NamedNumeric
        n75 = Unbundle By Name(w176) -> ("Control References.Components to Build"=w183:refnum<vi>, "View Type"=w169:T2, "Build Analyzer"=w168:refnum<class "Build Analyzer.lvclass">)
        n76 = case shown="\"Component View\", Default" w169 {
          tunnel: [w188 w192] -> w180
          tunnel: w168 -> [w187 w191]
          tunnel: w167 -> [w186 w190]
          tunnel: [w185 w189] -> w172
          frame "Component View", Default {
            n77 = property class="Build Analyzer"(reference=w187, error in=w186) -> (error out=w185:errorcluster, "Accessors:Comp Product To Unique Name"=w188:variant)  [unwired: 1 out]
          }
          frame "Export View" {
            n78 = property class="Build Analyzer"(reference=w191, error in=w190) -> (error out=w189:errorcluster, "Accessors:Export Product To Unique Name"=w192:variant)  [unwired: 1 out]
          }
        }
        n79 = property on="Property Node" class="Arr (strict)"(reference=w183, "Value"=u16[] []) -> (error out=w175:errorcluster, "Array Element"=w182:refnum<vi>)  [unwired: 1 in, 1 out]
        n80 = Get Variant Attribute(Variant=w180, error in=w172) -> (names=w179:string[], error out=w170:errorcluster)  [unwired: 2 in, 2 out]
        n81 = To More Specific Class(target class=w184, reference=w182, error in=w175) -> (specific class reference=w181:refnum<vi>, error out=w174:errorcluster)
        n82 = Sort 1D Array(array=w179) -> (sorted array=w178:string[])
        n83 = Bundle By Name(cluster=w176, "Buildable Components"=w178) -> (w177:T6)
        n84 = property on="Property Node" class="NmdNum"(reference=w181, error in=w174, "Strings []"=w178) -> (error out=w171:errorcluster)  [unwired: 1 out]
        n85 = Merge Errors(w170, w171) -> (w173:errorcluster)
      }
      frame "Pass Build Analysis" {
        n86 = Variant To Data(error in=w196, type=refnum<class "Build Analyzer.lvclass"> refnum ("Build Analyzer"), Variant=w197) -> (data=w193:refnum<class "Build Analyzer.lvclass">, error out=w195:errorcluster)
        n87 = Bundle By Name(cluster=w199, "Build Analyzer"=w193) -> (w194:T6)
      }
      frame "Generate Ordered List" {
        n88 = Unbundle By Name(w220) -> ("View Type"=w202:T2, "Build Analyzer"=w203:refnum<class "Build Analyzer.lvclass">, "Buildable Components"=w209:string[], "Components to Build"=w208:u16[], "Build Type"=w219:T5)
        n89 = for {
          tunnel: w209 -> [w231]
          tunnel: w208 -> [w230] mode=indexing
          tunnel: [w229] -> w205 mode=concatenating
          shift-right: [w226] -> w204
          shift-left: w203 -> [w227]
          tunnel: w202 -> [w225]
          n90 = Index Array(array=w231, index=w230) -> (element=w228:string)
          n91 = case shown="\"Component View\"" w225 {
            tunnel: [w232 w240] -> w229
            tunnel: w228 -> [w233 w238]
            tunnel: w227 -> [w234 w236]
            tunnel: [w234 w235] -> w226
            frame "Export View", Default {
              n92 = Build Array(w233) -> (w232:string[])
            }
            frame "Component View" {
              n93 = call "Get Component by Product Name.vi"("Build Analyzer in"=w236, "Component's Product Name"=w238) -> ("Build Analyzer out"=w235:refnum<class "Build Analyzer.lvclass">, "Component"=w237:refnum<class "Component.lvclass">)  [unwired: 10 in, 2 out]
              n94 = call "Get All Exports.vi"("Component in"=w237) -> ("Exports"=w239:refnum<class "Export.lvclass">[])  [unwired: 13 in, 1 out]
              n95 = for {
                tunnel: [w242] -> w240 mode=indexing
                tunnel: w239 -> [w241] mode=indexing
                n96 = property class="Export"(reference=w241) -> ("Accessors:Product Name"=w242:string)  [unwired: 1 in, 2 out]
              }
            }
          }
        }
        n97 = call "Hierarchy To Build Order.vi"("Build Analyzer in"=w204, "Export Product Names to build"=w205, "Build Type"=w219) -> ("Ordered Exports"=w200:refnum<class "Export.lvclass">[], "error out"=w207:errorcluster)  [unwired: 10 in, 1 out]
        n98 = for {
          tunnel: w200 -> [w224] mode=indexing
          tunnel: [w223] -> w218 mode=indexing
          shift-right: [w222] -> w206
          shift-left: w207 -> [w221]
          n99 = property class="Export"(reference=w224, error in=w221) -> (error out=w222:errorcluster, "Accessors:Product Name"=w223:string)  [unwired: 1 out]
        }
        n100 = Bundle By Name(cluster=w220, "Export Build Order"=w200) -> (w201:T6)
        n101 = Array To Spreadsheet String(delimiter (Tab)="\n", array=w218, 3:"" ("format string")) -> (spreadsheet string=w214:string)
        n102 = call-poly "Enqueue Message.vi"("error in (no error)"=w206, "Message Data"=w200, "Message"="New Ordered Exports Available", "Message Queue"=w212) -> ("error out"=w210:errorcluster)  [unwired: 6 in, 1 out]
        n103 = Format Into String(format string="The following exports will be created in the listed order:\n\n%s ", w214) -> (resulting string=w213:string)  [unwired: 2 in, 1 out]
        n104 = local write "Status"(w213) -> ()
      }
      frame "Update Selection View Type" {
        n105 = Variant To Data(error in=w253, type=Organizational_Types_View."Export View" ("Component \\ Export View 2"), Variant=w254) -> (data=w251:T2, error out=w250:errorcluster)
        n106 = call-poly "Enqueue Message.vi"("error in (no error)"=w250, "Message"="Populate Components To Build", "Message Queue"=w248) -> ("error out"=w246:errorcluster, "dup Message Queue"=w247:refnum<queue>)  [unwired: 7 in]
        n107 = call-poly "Enqueue Message.vi"("error in (no error)"=w246, "Message Data"=u16[] [], "Message"="Update Components To Build", "Message Queue"=w247) -> ("error out"=w245:errorcluster)  [unwired: 6 in, 1 out]
        n108 = Bundle By Name(cluster=w256, "View Type"=w251) -> (w255:T6)
      }
      frame "---Execute Build---" {
      }
      frame "Init Build" {
        n109 = Unbundle By Name(w282) -> ("Export Build Order"=w276:refnum<class "Export.lvclass">[], "Control References.Abort"=w267:refnum<vi>, "Control References.Shutdown"=w274:refnum<vi>, "Control References.Back"=w273:refnum<vi>, "Control References.Next"=w272:refnum<vi>, "Control References.Email Behavior Reference"=w271:refnum<vi>, "Control References.Sync Action"=w265:refnum<vi>, "Control References.Auto Submit Behavior"=w262:refnum<vi>, "Control References.Email Address"=w261:refnum<vi>, "Control References.Outgoing Mail Server"=w260:refnum<vi>, "Control References.Sender's Email Address"=w259:refnum<vi>)
        n110 = Build Array(w267) -> (w266:refnum<vi>[])
        n111 = Build Array(w274, w273, w272, w271, w265, w262, w261, w260, w259) -> (w269:refnum<vi>[])
        n112 = for {
          tunnel: [w284] -> w275 mode=indexing
          tunnel: w276 -> [w283] mode=indexing
          n113 = property class="Export"(reference=w283) -> ("Accessors:Product Name"=w284:string)  [unwired: 1 in, 2 out]
        }
        n114 = call "Set Enable State on Multiple Controls.vi"("Control References"=w266) -> ("error out"=w263:errorcluster)  [unwired: 13 in, 1 out]
        n115 = call "Set Enable State on Multiple Controls.vi"("Control References"=w269, "State"=T12."Disabled and Grayed Out" ("Disabled")) -> ("error out"=w270:errorcluster)  [unwired: 12 in, 1 out]
        n116 = local write "Status"("Press \"Abort\" to stop after the current build completes." ("Status")) -> ()
        n117 = local write "Build Phase"(T4."Build Status" ("Build Phase")) -> ()
        n118 = Merge Errors(w263, w270) -> (w264:errorcluster)
        n119 = property on="Exports" class="LstBox (strict)"("Value"=-1 ("Exports"), "Active Row"=-2 ("Active Row:Active Row Number"), "CellBG"=u32 16448250, "Item Names"=w275) -> ()  [unwired: 2 in, 2 out]
      }
      frame "Pre Build Check" {
        n120 = Unbundle By Name(w296) -> ("Control References.Abort"=w286:refnum<vi>, "Control References.Shutdown"=w292:refnum<vi>, "Control References.Back"=w291:refnum<vi>, "Control References.Next"=w290:refnum<vi>, "Control References.Component \\ Export View Reference"=w289:refnum<vi>)
        n121 = Build Array(w292, w291, w290, w289) -> (w288:refnum<vi>[])
        n122 = Build Array(w286) -> (w285:refnum<vi>[])
        n123 = call "Set Enable State on Multiple Controls.vi"("Control References"=w285, "State"=T12."Disabled" ("Disabled")) -> ()  [unwired: 12 in, 2 out]
        n124 = call "Set Enable State on Multiple Controls.vi"("Control References"=w288, "State"=T12."Disabled and Grayed Out" ("Disabled")) -> ("error out"=w287:errorcluster)  [unwired: 12 in, 1 out]
        n125 = local write "Status"("Ruinning commit checks.\nCleaning previous exports and making new exports.\n" ("Status")) -> ()
      }
      frame "Pre Build Commit Readiness Failure" {
        n126 = Variant To Data(type="" ("spreadsheet string"), Variant=w302) -> (data=w297:string, error out=w301:errorcluster)  [unwired: 1 in]
        n127 = Format Into String(format string="One or more checks for succesfully committing builds failed. Aborting the build \n%s", w297) -> (resulting string=w299:string)  [unwired: 2 in, 1 out]
        n128 = local write "Status"(w299) -> ()
      }
      frame "Update Build Marker" {
        n129 = Variant To Data(error in=w308, type=u32 0 ("Build Marker"), Variant=w309) -> (data=w304:u32, error out=w307:errorcluster)
        n130 = property on="Exports" class="LstBox (strict)"("Active Row"=w304, "CellBG"=u32 16773632) -> ()  [unwired: 2 in, 2 out]
        n131 = Bundle By Name(cluster=w311, "Build Marker"=w304) -> (w305:T6)
      }
      frame "Final Build Status" {
        n132 = Variant To Data(error in=w312, type=errorcluster {"status"=FALSE, "code"=0, "source"=""} ("error out"), Variant=w316) -> (data=w314:errorcluster, error out=w313:errorcluster)
        n133 = Unbundle By Name(w318) -> ("Build Marker"=w317:u32)
        n134 = Select(t=u32 16711735, s=w314, f=u32 1244948) -> (s? t:f=w319:u32)
        n135 = property on="Exports" class="LstBox (strict)"("Active Row"=w317, "CellBG"=w319) -> ()  [unwired: 2 in, 2 out]
      }
      frame "Build Complete" {
        w335 = -2 ("Value")
        w332 = T12."Enabled" ("Disabled")
        n136 = Variant To Data(error in=w345, type=T13 {"Ordered Exports"=[], "Build Groups Folder"=path ""} ("input cluster"), Variant=w346) -> (data=w328:T13, error out=w330:errorcluster)
        n137 = Unbundle By Name(w328) -> ("Build Groups Folder"=w324:path, "Ordered Exports"=w327:refnum<class "Export.lvclass">[])
        n138 = local write "Build Phase"(T4."Build Results" ("Build Phase")) -> ()
        n139 = for {
          tunnel: w327 -> [w358] mode=indexing
          tunnel: [w354] -> w323 mode=indexing if=w351
          tunnel: [w354] -> w342 mode=indexing if=w357
          n140 = property class="Export"(reference=w358) -> ("Accessors:Product Name"=w356:string, "Accessors:Built Version"=w355:string, "Accessors:Merged Errors"=w352:errorcluster)  [unwired: 1 in, 2 out]
          n141 = Unbundle By Name(w352) -> ("status"=w351:bool)
          n142 = Not(x=w352) -> (.not. x?=w357:bool)
          n143 = Concatenate Strings(w356, " - " ("string"), w355) -> (w354:string)
        }
        n144 = Bundle By Name(cluster=w350, "Build Groups Folder"=w324, "Build Results"=w327) -> (w349:T6)
        n145 = Unbundle By Name(w349) -> ("Control References.Shutdown"=w333:refnum<vi>, "Control References.Back"=w348:refnum<vi>, "Control References.Next"=w347:refnum<vi>, "Control References.Failed Builds"=w344:refnum<vi>, "Control References.Successful Builds"=w343:refnum<vi>)
        n146 = property class="LstBox (strict)"(reference=w344, "Item Names"=w323, "Value"=w335) -> (error out=w339:errorcluster)  [unwired: 1 in, 1 out]
        n147 = property class="LstBox (strict)"(reference=w343, "Item Names"=w342, "Value"=w335) -> (error out=w338:errorcluster)  [unwired: 1 in, 1 out]
        n148 = property class="Bool"(reference=w348, "DisabledEnum"=w332, "BoolText.Text"="Delete Exports" ("Boolean Text.Text")) -> (error out=w341:errorcluster)  [unwired: 1 in, 1 out]
        n149 = property class="Bool"(reference=w347, "DisabledEnum"=w332, "BoolText.Text"="Commit" ("Boolean Text.Text")) -> (error out=w340:errorcluster)  [unwired: 1 in, 1 out]
        n150 = property class="Bool"(reference=w333, "DisabledEnum"=w332) -> (error out=w331:errorcluster)  [unwired: 1 in, 1 out]
        n151 = Format Into String(format string="Build Complete. Select items to see details.\nThe group of build exports may be found at:\n%s" ("Status"), w324) -> (resulting string=w326:string)  [unwired: 2 in, 1 out]
        n152 = local write "Status"(w326) -> ()
        n153 = Merge Errors(w330, w331, w341, w340, w339, w338) -> (w322:errorcluster)
      }
      frame "Send Email" {
        n154 = Unbundle By Name(w364) -> ("Build Results"=w363:refnum<class "Export.lvclass">[])
        n155 = Variant To Data(type=Email_Behavior."Do Not Email" ("Email Behavior 2"), Variant=w362) -> (data=w360:T1, error out=w359:errorcluster)  [unwired: 1 in]
        n156 = case shown="Default" w360 {
          selector: w360 -> [_ w365]
          tunnel: w363 -> [_ w371]
          frame "Do Not Email" {
          }
          frame Default {
            n157 = for {
              tunnel: w371 -> [w449] mode=indexing
              tunnel: "Export\n\n%s\n\nof Component \n\n%s\n\nfailed to build with the following error:\n\nCode: %d\n\nSource:\n%s" ("format string") -> [w448]
              tunnel: [w443] -> w373 mode=indexing if=w442
              tunnel: [w442] -> w369 if=w442
              tunnel: [w440] -> w370 mode=indexing
              n158 = property class="Export"(reference=w449) -> ("Accessors:Built Version"=w438:string, "Accessors:Product Name"=w439:string, "Accessors:Owning Component's Product Name"=w447:string, "Accessors:Merged Errors"=w446:errorcluster)  [unwired: 1 in, 2 out]
              n159 = Unbundle By Name(w446) -> ("code"=w445:i32, "source"=w444:string, "status"=w442:bool)
              n160 = Format Into String(format string=w448, w439, w447, w445, w444) -> (resulting string=w443:string)  [unwired: 2 in, 1 out]
              n161 = Concatenate Strings(w439, "-" ("string"), w438) -> (w440:string)
            }
            n162 = Array Size(array=w371) -> (size(s)=w374:i32)
            n163 = case shown="False" w369 {
              tunnel: w373 -> [w415 _]
              tunnel: w374 -> [w412 _]
              tunnel: [w408 w428] -> w367
              tunnel: [w407 w427] -> w366
              tunnel: w370 -> [_ w426]
              frame True {
                n164 = String To IP() -> (0:w421:u32)  [unwired: 1 in]
                n165 = Array Size(array=w415) -> (size(s)=w413:i32)
                n166 = Array To Spreadsheet String(delimiter (Tab)="----------\n", array=w415, 3:"" ("format string")) -> (spreadsheet string=w418:string)
                n167 = IP To String(1:FALSE ("dot notation? (F)"), 2:w421) -> (0:w416:string)
                n168 = IP To String(1:TRUE ("dot notation? (F)"), 2:w421) -> (0:w410:string)
                n169 = call <vilib>:"Trim Whitespace.vi"("string"=w418) -> ("trimmed string"=w409:string)  [unwired: 1 in]
                n170 = Format Into String(format string="The follwoing errors were generated during build on computer named\n%s\nat\nIP Address: %s\n\n%s ", w416, w410, w409) -> (resulting string=w408:string)  [unwired: 2 in, 1 out]
                n171 = Format Into String(format string="%d Build Errors Out of %d Attempted Exports on Computer\"%s\", IP Address \"%s\"" ("Subject"), w413, w412, w416, w410) -> (resulting string=w407:string)  [unwired: 2 in, 1 out]
              }
              frame False {
                n172 = String To IP() -> (0:w436:u32)  [unwired: 1 in]
                n173 = Array Size(array=w426) -> (size(s)=w432:i32)
                n174 = Array To Spreadsheet String(delimiter (Tab)="\n" ("format string"), array=w426, 3:"" ("format string")) -> (spreadsheet string=w434:string)
                n175 = IP To String(1:FALSE ("dot notation? (F)"), 2:w436) -> (0:w433:string)
                n176 = IP To String(1:TRUE ("dot notation? (F)"), 2:w436) -> (0:w430:string)
                n177 = call <vilib>:"Trim Whitespace.vi"("string"=w434) -> ("trimmed string"=w429:string)  [unwired: 1 in]
                n178 = Format Into String(format string="All components were sucessfully built:\n%s\nat\nIP Address: %s\n\n%s ", w433, w430, w429) -> (resulting string=w428:string)  [unwired: 2 in, 1 out]
                n179 = Format Into String(format string="No Build Errors. %d Built Exports on Computer\"%s\", IP Address \"%s\"" ("Subject"), w432, w433, w430) -> (resulting string=w427:string)  [unwired: 2 in, 1 out]
              }
            }
            n180 = case shown="\"Email On All Successfully Built\"" w365 {
              tunnel: w369 -> [_ w375 w377 _]
              tunnel: [_ w375 w376 TRUE ("status")] -> w368
              frame "Do Not Email", Default {
              }
              frame "Email On Any Failure" {
              }
              frame "Email On All Successfully Built" {
                n181 = Not(x=w377) -> (.not. x?=w376:bool)
              }
              frame "Email On Success OR Failure" {
              }
            }
            n182 = case shown="True" w368 {
              tunnel: w367 -> [_ w387]
              tunnel: w366 -> [_ w388]
              frame False {
                # "Don't Send Email"
              }
              frame True {
                # "Send Email"
                n183 = for {
                  tunnel: "Email Address" -> [w406] mode=indexing
                  tunnel: [w405] -> w389 mode=indexing
                  n184 = call <vilib>:"Trim Whitespace.vi"("string"=w406) -> ("trimmed string"=w405:string)  [unwired: 1 in]
                }
                n185 = Format Into String(format string=":%d", initial string="Outgoing Mail Server", u16 25 ("input 1")) -> (resulting string=w385:string)  [unwired: 1 in, 1 out]
                n186 = call <vilib>:"Open Handle.vi"("server address"=w385, "from"="Sender's Email Address") -> ("handle out"=w398:T14, "error out"=w397:errorcluster)  [unwired: 12 in]
                n187 = call <vilib>:"Set Recipients.vi"("handle in"=w398, "to"=w389, "error in (no error)"=w397) -> ("handle out"=w396:T14, "error out"=w395:errorcluster)  [unwired: 11 in]
                n188 = call-poly <vilib>:"Set Message.vi"("handle in"=w396, "subject"=w388, "plain text message"=w387, "error in (no error)"=w395) -> ("handle out"=w393:T14, "error out"=w394:errorcluster)  [unwired: 10 in]
                n189 = call <vilib>:"Send.vi"("handle in"=w393, "error in (no error)"=w394) -> ("handle out"=w391:T14, "invalid recipients"=w381:string[], "error out"=w392:errorcluster)  [unwired: 11 in]
                n190 = Array Size(array=w381) -> (size(s)=w380:i32)
                n191 = call <vilib>:"Close Handle.vi"("handle in"=w391, "error in (no error)"=w392) -> ("error out"=w379:errorcluster)  [unwired: 12 in, 1 out]
                n192 = case shown="Default" w380 {
                  tunnel: w381 -> [_ w399]
                  frame 0 {
                  }
                  frame Default {
                    n193 = Array To Spreadsheet String(delimiter (Tab)="\n", array=w399, 3:"" ("format string")) -> (spreadsheet string=w403:string)
                    n194 = Format Into String(format string="Invalid Receipients Specified:\n %s" ("message"), w403) -> (resulting string=w400:string)  [unwired: 2 in, 1 out]
                    n195 = One Button Dialog(message=w400) -> ()  [unwired: 1 in, 1 out]
                  }
                }
                n196 = call <vilib>:"Clear Errors.vi"("error in (no error)"=w379) -> ()  [unwired: 5 in, 2 out]
              }
            }
          }
        }
      }
      frame "Post Build" {
      }
      frame "Abort" {
        n197 = Unbundle By Name(w456) -> ("Control References.Abort"=w455:refnum<vi>)
        n198 = local write "Status"("Aborting after current build completes..." ("Status")) -> ()
        n199 = Build Array(w455) -> (w454:refnum<vi>[])
        n200 = call "Set Enable State on Multiple Controls.vi"("Control References"=w454, "State"=T12."Disabled and Grayed Out" ("Disabled")) -> ("error out"=w452:errorcluster)  [unwired: 12 in, 1 out]
      }
      frame "Select All" {
        n201 = Unbundle By Name(w467) -> ("Control References.Front Panel"=w460:refnum<vi>, "Build Analyzer"=w476:refnum<class "Build Analyzer.lvclass">, "Build Type"=w477:T5, "Buildable Components"=w472:string[], "Control References.Next"=w470:refnum<vi>)
        n202 = flat-sequence {
          tunnel: w472 -> [w481]
          tunnel: w476 -> [w482]
          tunnel: w477 -> [w483]
          tunnel: [w483] -> w464
          tunnel: [w482] -> w463
          tunnel: [w481] -> w462
          tunnel: w460 -> [w480]
          tunnel: [w479] -> w458
          tunnel: [w484] -> w474
          tunnel: w467 -> [w495]
          tunnel: [w491] -> w465
          tunnel: w464 -> [w502]
          tunnel: w463 -> [w489]
          tunnel: w462 -> [w486]
          tunnel: [w493] -> w461
          tunnel: [w490] -> w459
          tunnel: w458 -> [w490]
          tunnel: [w518] -> w466
          tunnel: w461 -> [w518]
          tunnel: w459 -> [w517]
          frame #0 {
            n203 = property class="Pnl"(reference=w480, "DeferPanUpdts"=TRUE ("Defer Panel Updates")) -> (reference out=w479:refnum<vi>)  [unwired: 1 in, 1 out]
          }
          frame #1 {
            n204 = for {
              tunnel: [w508] -> w487 mode=concatenating
              shift-right: [w504] -> w488
              shift-left: w489 -> [w505]
              tunnel: w486 -> [w503] mode=indexing
              n205 = call "Get Component by Product Name.vi"("Build Analyzer in"=w505, "Component's Product Name"=w503) -> ("Build Analyzer out"=w504:refnum<class "Build Analyzer.lvclass">, "Component"=w506:refnum<class "Component.lvclass">)  [unwired: 10 in, 2 out]
              n206 = call "Get All Exports.vi"("Component in"=w506) -> ("Exports"=w507:refnum<class "Export.lvclass">[])  [unwired: 13 in, 1 out]
              n207 = for {
                tunnel: [w510] -> w508 mode=indexing
                tunnel: w507 -> [w509] mode=indexing
                n208 = property class="Export"(reference=w509) -> ("Accessors:Product Name"=w510:string)  [unwired: 1 in, 2 out]
              }
            }
            n209 = Array Size(array=w486) -> (size(s)=w485:i32)
            n210 = for {
              N: w485 -> [_]
              tunnel: [w515] -> w494 mode=indexing
              i -> [w515]
            }
            n211 = call "Hierarchy To Build Order.vi"("Build Analyzer in"=w488, "Export Product Names to build"=w487, "Build Type"=w502) -> ("Ordered Exports"=w484:refnum<class "Export.lvclass">[], "error out"=w492:errorcluster)  [unwired: 10 in, 1 out]
            n212 = for {
              tunnel: w484 -> [w514] mode=indexing
              tunnel: [w513] -> w501 mode=indexing
              shift-right: [w511] -> w491
              shift-left: w492 -> [w512]
              n213 = property class="Export"(reference=w514, error in=w512) -> (error out=w511:errorcluster, "Accessors:Product Name"=w513:string)  [unwired: 1 out]
            }
            n214 = Array To Spreadsheet String(delimiter (Tab)=",\n", array=w501, 3:"" ("format string")) -> (spreadsheet string=w497:string)
            n215 = Format Into String(format string="The following exports will be created in the listed order:\n%s ", w497) -> (resulting string=w496:string)  [unwired: 2 in, 1 out]
            n216 = Bundle By Name(cluster=w495, "Export Build Order"=w484, "Components to Build"=w494) -> (w493:T6)
            n217 = local write "Components to build"(w494) -> ()
            n218 = local write "Status"(w496) -> ()
          }
          frame #2 {
            n219 = property class="Pnl"(reference=w517, "DeferPanUpdts"=FALSE ("Defer Panel Updates")) -> ()  [unwired: 1 in, 2 out]
          }
        }
        n220 = property class="Bool"(reference=w470, error in=w465, "DisabledEnum"=T12."Enabled" ("Disabled")) -> (error out=w469:errorcluster)  [unwired: 1 out]
        n221 = call-poly "Enqueue Message.vi"("error in (no error)"=w469, "Message Data"=w474, "Message"="New Ordered Exports Available", "Message Queue"=w475) -> ("error out"=w468:errorcluster)  [unwired: 6 in, 1 out]
      }
      frame "Select None" {
        w523 = u16[] [] items=["agilent 3631a", "agilent e4980 driver", "ap27xx", "apx5xx", "apx5xx vendor api", "audio driver palette installer", "cbt", "clive", "cmw", "database logging teststand api", "database logging teststand api - hack", "datalogging", "db utility", "digital driver palette installer", "digital interface", "dmm class", "dmm driver palette installer", "email text result", "email text result teststand api", "email text result teststand api - hack", "g3 teststand customizations", "hsdio serial interface", "hsdio teststand api", "hsdio teststand api - hack", "i2c digital waveform", "instek psmx", "instrument driver palette installer", "iteration tools", "iteration tools teststand api", "iteration tools teststand api - hack", "keithley 2000", "keithley 24xx", "keithley 26xx", "ni dc power", "ni-dmm", "ni-dsa", "ni-scope", "power supply", "power supply driver palette installer", "project instantiation tool", "promira", "quickdrop plugins", "reusables", "rf driver palette installer", "rssmb 100a", "scope driver palette installer", "signal generator driver palette installer", "silicon delta", "tektronix afg2k 3k", "tektronix rsa 6100 driver", "tektronix scope", "test instantiation tool", "thermal driver palette installer", "vicomponentbuilder"] ("Components to build")
        n222 = Unbundle By Name(w522) -> ("Control References.Next"=w521:refnum<vi>)
        n223 = Bundle By Name(cluster=w522, "Components to Build"=w523) -> (w524:T6)
        n224 = local write "Components to build"(w523) -> ()
        n225 = local write "Status"("No Components Selected to build" ("Status")) -> ()
        n226 = property class="Bool"(reference=w521, "DisabledEnum"=T12."Disabled and Grayed Out" ("Disabled")) -> (error out=w519:errorcluster)  [unwired: 1 in, 1 out]
      }
      frame "Update Components To Build" {
        w539 = u16[] [] items=["agilent 3631a", "agilent e4980 driver", "ap27xx", "apx5xx", "apx5xx vendor api", "audio driver palette installer", "cbt", "clive", "cmw", "database logging teststand api", "database logging teststand api - hack", "datalogging", "db utility", "digital driver palette installer", "digital interface", "dmm class", "dmm driver palette installer", "email text result", "email text result teststand api", "email text result teststand api - hack", "g3 teststand customizations", "hsdio serial interface", "hsdio teststand api", "hsdio teststand api - hack", "i2c digital waveform", "instek psmx", "instrument driver palette installer", "iteration tools", "iteration tools teststand api", "iteration tools teststand api - hack", "keithley 2000", "keithley 24xx", "keithley 26xx", "ni dc power", "ni-dmm", "ni-dsa", "ni-scope", "power supply", "power supply driver palette installer", "project instantiation tool", "promira", "quickdrop plugins", "reusables", "rf driver palette installer", "rssmb 100a", "scope driver palette installer", "signal generator driver palette installer", "silicon delta", "tektronix afg2k 3k", "tektronix rsa 6100 driver", "tektronix scope", "test instantiation tool", "thermal driver palette installer", "vicomponentbuilder"] ("Components to build")
        n227 = Variant To Data(type=w539, Variant=w538) -> (data=w533:u16[], error out=w529:errorcluster)  [unwired: 1 in]
        n228 = Unbundle By Name(w535) -> ("Control References.Next"=w528:refnum<vi>)
        n229 = Empty Array?(array=w533) -> (empty?=w534:bool)
        n230 = Select(t=T12."Disabled and Grayed Out" ("Disabled"), s=w534, f=T12."Enabled" ("Disabled")) -> (s? t:f=w526:T12)
        n231 = Build Array(w528) -> (w527:refnum<vi>[])
        n232 = call "Set Enable State on Multiple Controls.vi"("Control References"=w527, "State"=w526) -> ()  [unwired: 12 in, 2 out]
        n233 = call-poly "Enqueue Message.vi"("error in (no error)"=w529, "Message"="Generate Ordered List", "Message Queue"=w536) -> ("error out"=w530:errorcluster)  [unwired: 7 in, 1 out]
        n234 = Bundle By Name(cluster=w535, "Components to Build"=w533) -> (w537:T6)
      }
      frame "Update Selected Successful Build" {
        n235 = Variant To Data(type=0, Variant=w550) -> (data=w544:i32, error out=w548:errorcluster)  [unwired: 1 in]
        n236 = Unbundle By Name(w547) -> ("Control References.Successful Builds"=w546:refnum<vi>)
        n237 = property class="LstBox (strict)"(reference=w546) -> ("Item Names"=w545:string[])  [unwired: 1 in, 2 out]
        n238 = Index Array(array=w545, index=w544) -> (element=w542:string)
        n239 = Format Into String(format string="No build errors for component \n%s", w542) -> (resulting string=w541:string)  [unwired: 2 in, 1 out]
        n240 = local write "Status"(w541) -> ()
      }
      frame "Update Selected Failed Build" {
        n241 = Variant To Data(type=0, Variant=w565) -> (data=w559:i32, error out=w563:errorcluster)  [unwired: 1 in]
        n242 = Unbundle By Name(w562) -> ("Build Results"=w558:refnum<class "Export.lvclass">[], "Control References.Failed Builds"=w561:refnum<vi>)
        n243 = property class="LstBox (strict)"(reference=w561) -> ("Item Names"=w560:string[])  [unwired: 1 in, 2 out]
        n244 = Index Array(array=w560, index=w559) -> (element=w554:string)
        n245 = for {
          tunnel: w558 -> [w570] mode=indexing
          tunnel: w554 -> [w569]
          tunnel: [w567] -> w557
          stop <- w568 stop-if-true
          n246 = property class="Export"(reference=w570) -> (reference out=w567:refnum<class "Export.lvclass">, "Accessors:Product Name"=w566:string)  [unwired: 1 in, 1 out]
          n247 = Equal?(x=w566, y=w569) -> (x = y?=w568:bool)
        }
        n248 = call "Read Export Operation Errors.vi"("Export in"=w557) -> ("Export Operation Errors"=w555:errorcluster)  [unwired: 8 in, 2 out]
        n249 = Unbundle By Name(w555) -> ("code"=w553:i32, "source"=w552:string)
        n250 = Format Into String(format string="Component %s had the following build errors:\nCode %d\n%s", w554, w553, w552) -> (resulting string=w551:string)  [unwired: 2 in, 1 out]
        n251 = local write "Status"(w551) -> ()
      }
      frame "---Commit---" {
      }
      frame "Commit" {
        n252 = Unbundle By Name(w579) -> ("Control References.Back"=w576:refnum<vi>, "Control References.Next"=w575:refnum<vi>)
        n253 = Build Array(w576, w575) -> (w577:refnum<vi>[])
        n254 = call "Set Enable State on Multiple Controls.vi"("Control References"=w577, "State"=T12."Disabled and Grayed Out" ("Disabled")) -> ("error out"=w574:errorcluster)  [unwired: 12 in, 1 out]
        n255 = local write "Status"("Running commit behavior for each successfully built export... Please wait." ("Status")) -> ()
      }
      frame "Commit Readiness Failure" {
        n256 = Variant To Data(type="" ("spreadsheet string"), Variant=w585) -> (data=w580:string, error out=w584:errorcluster)  [unwired: 1 in]
        n257 = Format Into String(format string="The check for succesful commit failed:\n%s", w580) -> (resulting string=w582:string)  [unwired: 2 in, 1 out]
        n258 = local write "Status"(w582) -> ()
      }
      frame "Submission Status Val Change" {
        n259 = Unbundle By Name(w591) -> ("Build Results"=w590:refnum<class "Export.lvclass">[])
        n260 = Variant To Data(type=0, Variant=w595) -> (data=w592:i32, error out=w593:errorcluster)  [unwired: 1 in]
        n261 = Index Array(array=w590, index=w592) -> (element=w589:refnum<class "Export.lvclass">)
        n262 = call "Read Export Operation Errors.vi"("Export in"=w589) -> ("Export Operation Errors"=w587:errorcluster)  [unwired: 8 in, 2 out]
        n263 = case shown="Error" w587 {
          selector: w587 -> [_ w597]
          tunnel: ["Submitted Successfully." w598] -> w588
          frame No Error {
          }
          frame Error {
            n264 = Unbundle By Name(w597) -> ("code"=w600:i32, "source"=w599:string)
            n265 = Format Into String(format string="Code:%d\nStatus: %s", w600, w599) -> (resulting string=w598:string)  [unwired: 2 in, 1 out]
          }
        }
        n266 = local write "Status"(w588) -> ()
      }
      frame "Commit Complete" {
        w612 = u16[] [] ("Components to build")
        n267 = Unbundle By Name(w611) -> ("Control References.Components to Build"=w603:refnum<vi>, "Build Results"=w605:refnum<class "Export.lvclass">[])
        n268 = for {
          tunnel: w605 -> [w616] mode=indexing
          tunnel: [w614] -> w604 mode=indexing if=w614
          n269 = property class="Export"(reference=w616) -> ("Accessors:Merged Errors"=w615:errorcluster)  [unwired: 1 in, 2 out]
          n270 = Unbundle By Name(w615) -> ("status"=w614:bool)
        }
        n271 = Build Array(w603) -> (w602:refnum<vi>[])
        n272 = call "Set Enable State on Multiple Controls.vi"("Control References"=w602) -> ()  [unwired: 13 in, 2 out]
        n273 = Empty Array?(array=w604) -> (empty?=w609:bool)
        n274 = Bundle By Name(cluster=w611, "Components to Build"=w612) -> (w613:T6)
        n275 = local write "Components to build"(w612) -> ()
        n276 = Select(t="Exports Removed and Post Submit successfuly executed. Select Exports to build." ("Status"), s=w609, f="Failed to submit, clean, or post submit at least one export. Select Export to see error. \nPlease shutdown the builder and fix all errors " ("Status")) -> (s? t:f=w608:string)
        n277 = local write "Status"(w608) -> ()
      }
      frame "Exports Cleaned" {
        w632 = u16[] [] ("Components to build")
        n278 = Variant To Data(error in=w629, type=refnum<class "Export.lvclass">[] [] ("Ordered Exports"), Variant=w630) -> (data=w626:refnum<class "Export.lvclass">[], error out=w628:errorcluster)
        n279 = for {
          tunnel: w626 -> [w638] mode=indexing
          tunnel: [w636] -> w624 mode=indexing
          n280 = property class="Export"(reference=w638) -> ("Accessors:Product Name"=w637:string, "Accessors:Built Version"=w635:string)  [unwired: 1 in, 2 out]
          n281 = Concatenate Strings(w637, " - " ("string"), w635) -> (w636:string)
        }
        n282 = Unbundle By Name(w631) -> ("Control References.Components to Build"=w618:refnum<vi>)
        n283 = Array To Spreadsheet String(delimiter (Tab)="\n", array=w624, 3:"" ("format string")) -> (spreadsheet string=w622:string)
        n284 = call <vilib>:"Trim Whitespace.vi"("string"=w622) -> ("trimmed string"=w621:string)  [unwired: 1 in]
        n285 = Build Array(w618) -> (w617:refnum<vi>[])
        n286 = Bundle By Name(cluster=w631, "Build Results"=w626, "Components to Build"=w632) -> (w633:T6)
        n287 = local write "Components to build"(w632) -> ()
        n288 = Format Into String(format string="The follwoing exports were delete and  NOT submitted:\n%s " ("Status"), w621) -> (resulting string=w620:string)  [unwired: 2 in, 1 out]
        n289 = call "Set Enable State on Multiple Controls.vi"("Control References"=w617) -> ()  [unwired: 13 in, 2 out]
        n290 = local write "Status"(w620) -> ()
      }
      frame "Finished" {
        w646 = -2 ("Value")
        n291 = Unbundle By Name(w656) -> ("Control References.Outgoing Mail Server"=w640:refnum<vi>, "Control References.Sender's Email Address"=w641:refnum<vi>, "Control References.Auto Submit Behavior"=w642:refnum<vi>, "Control References.Email Address"=w643:refnum<vi>, "Control References.Email Behavior Reference"=w644:refnum<vi>, "Control References.Component \\ Export View Reference"=w645:refnum<vi>, "Control References.Back"=w651:refnum<vi>, "Control References.Submission Status"=w658:refnum<vi>)
        n292 = Variant To Data(type=refnum<class "Export.lvclass">[] [] ("Ordered Exports"), Variant=w660) -> (data=w655:refnum<class "Export.lvclass">[], error out=w648:errorcluster)  [unwired: 1 in]
        n293 = for {
          tunnel: w655 -> [w672] mode=indexing
          tunnel: [w668] -> w657 mode=indexing
          n294 = property class="Export"(reference=w672) -> ("Accessors:Product Name"=w671:string, "Accessors:Built Version"=w670:string)  [unwired: 1 in, 2 out]
          n295 = Concatenate Strings(w671, " - " ("string"), w670) -> (w668:string)
        }
        n296 = local write "Build Phase"(T4."Results" ("Build Phase")) -> ()
        n297 = Build Array(w640, w641, w642, w643, w644, w645) -> (w639:refnum<vi>[])
        n298 = call "Set Enable State on Multiple Controls.vi"("Control References"=w639) -> ()  [unwired: 13 in, 2 out]
        n299 = property class="LstBox (strict)"(reference=w658, "Item Names"=w657, "Active Row"=w646, "CellBG"=u32 16448250, "Value"=w646) -> (reference out=w653:refnum<vi>)  [unwired: 1 in, 1 out]
        n300 = property class="Bool"(reference=w651, "DisabledEnum"=T12."Enabled" ("Disabled"), "BoolText.Text"="Start Over" ("Boolean Text.Text")) -> ()  [unwired: 1 in, 2 out]
        n301 = for {
          tunnel: w655 -> [w662] mode=indexing
          tunnel: w653 -> [w667]
          i -> [w666]
          n302 = property class="Export"(reference=w662) -> ("Accessors:Merged Errors"=w661:errorcluster)  [unwired: 1 in, 2 out]
          n303 = Select(t=u32 16711680, s=w661, f=u32 6618880) -> (s? t:f=w665:u32)
          n304 = property class="LstBox (strict)"(reference=w667, "Active Row"=w666, "CellBG"=w665) -> ()  [unwired: 1 in, 2 out]
        }
        n305 = Bundle By Name(cluster=w656, "Build Results"=w655) -> (w654:T6)
      }
      frame "Exit" {
        # "Release the message queue reference"
        # "Exit - Exit the application."
        n306 = Release Queue(queue=w678, error in (no error)=w673) -> (error out=w675:errorcluster)  [unwired: 1 in, 2 out]
        n307 = Merge Errors(w675) -> (w674:errorcluster)
      }
      frame "Error" {
        # "Error - Check the error message data and respond accordingly. This message is sent by the \"Error Handler\" VIs at the end of each loop in this application."
        n308 = Variant To Data(error in=w690, type=errorcluster {"status"=FALSE, "code"=0, "source"=""} ("error constant"), Variant=w688) -> (data=w686:errorcluster, error out=w685:errorcluster)
        n309 = call <vilib>:"Simple Error Handler.vi"("error source (\" \")"="UI Manager" ("error source (\" \")"), "error in (no error)"=w686) -> ()  [unwired: 3 in, 5 out]
        n310 = call-poly "Enqueue Message.vi"("Priority Message? (F)"=TRUE, "Message"="Exit", "Message Queue"=w680) -> ("error out"=w684:errorcluster)  [unwired: 7 in, 1 out]
        n311 = Merge Errors(w684, w685) -> (w683:errorcluster)
      }
      frame Default {
        # "'Default' case only runs if there is a message that isn't defined in any of the other cases.  Output a programming error."
        n312 = xnode "Error Ring"("parameter 0"=w691) -> ("error out"=w692:errorcluster)
      }
      frame "---Update Local Data---" {
      }
      frame "Update Build Analyzer" {
        n313 = Variant To Data(type=refnum<class "Build Analyzer.lvclass"> refnum ("Build Analyzer"), Variant=w707) -> (data=w704:refnum<class "Build Analyzer.lvclass">, error out=w703:errorcluster)  [unwired: 1 in]
        n314 = Bundle By Name(cluster=w706, "Build Analyzer"=w704) -> (w705:T6)
      }
      frame "Update Build Type" {
        n315 = Variant To Data(type=T5."Bubble Up" ("Build Type"), Variant=w717) -> (data=w713:T5, error out=w710:errorcluster)  [unwired: 1 in]
        n316 = Bundle By Name(cluster=w715, "Build Type"=w713) -> (w714:T6)
        n317 = call-poly "Enqueue Message.vi"("error in (no error)"=w710, "Message"="Generate Ordered List", "Message Queue"=w712) -> ("error out"=w709:errorcluster)  [unwired: 7 in, 1 out]
      }
    }
    n318 = call "Error Handler - Message Handling Loop.vi"("error in (no error)"=w26, "Message Queue"=w24) -> ("dup error in"=w25:errorcluster)  [unwired: 8 in, 1 out]
  }
  n319 = while {
    tunnel: w19 -> [w722]
    tunnel: w11 -> [w726]
    shift-right: [w728] -> _
    shift-left: w15 -> [w729]
    tunnel: [w719] -> w17
    tunnel: w14 -> [w721]
    stop <- w727 stop-if-true
    # "Build Engine"
    n320 = call "Dequeue Message.vi"("error in (no error)"=w726, "Message Queue"=w722) -> ("error out"=w725:errorcluster, "Message Data"=w723:variant, "Message"=w724:string, "dup Message Queue"=w718:refnum<queue>)  [unwired: 6 in]
    n321 = case "Message Cases" shown="\"Build\"" w724 {
      selector: w724 -> [_ _ _ _ _ _ _ _ _ _ _ _ _ _ _ _ _ _ _ _ _ _ w1438]
      tunnel: w718 -> [w748 _ _ _ _ _ _ _ w960 w980 w992 w1047 _ w1153 w1163 _ w1170 w1218 w1235 _ _ w1428 _]
      tunnel: w725 -> [w731 _ w862 w878 w882 w894 w897 _ _ _ _ _ w1151 w1161 w1165 w1167 _ _ _ _ _ w1426 _]
      tunnel: [w746 w830 w869 w877 w882 w887 w895 w911 w959 w974 w986 w1039 w1151 w1161 w1165 w1167 w1171 w1216 w1223 w1372 w1404 w1417 w1439] -> w720
      tunnel: [w733 w836 w871 w873 w879 w893 w896 w904 w962 w979 w993 w1045 w1148 w1157 w1164 w1166 w1174 w1219 w1236 w1371 w1403 w1424 w1440] -> w728
      tunnel: w729 -> [w730 w826 w870 w875 w881 w893 w896 w903 w943 w979 w994 w1046 w1148 w1159 w1164 w1166 w1173 w1219 w1225 w1361 w1408 w1424 w1440]
      tunnel: [_ _ _ _ _ _ _ _ _ _ _ _ _ _ _ _ _ _ _ _ _ TRUE _] -> w727
      tunnel: w723 -> [_ _ _ w876 _ w892 _ w899 _ _ _ _ _ _ _ _ _ _ _ _ _ _ _]
      tunnel: w721 -> [_ w833 _ _ _ w884 _ w909 _ w977 _ w1040 w1150 _ _ _ w1172 _ _ w1373 w1407 _ _]
      frame "Initialize" {
        # "Initialize - Send separate messages to initialize the data and the front panel.  Bundle control references."
        n322 = Current VI's Path() -> (path=w739:path)
        n323 = Path to Array of Strings(0:w739) -> (2:w742:string[])  [unwired: 1 out]
        n324 = Search 1D Array(1D array=w742, element="Source") -> (index of element=w741:i32)  [unwired: 1 in]
        n325 = Split 1D Array(array=w742, index=w741) -> (first subarray=w740:string[])  [unwired: 1 out]
        n326 = Array of Strings to Path(0:w740) -> (2:w744:path)  [unwired: 1 in]
        n327 = Build Path(base path=w744, name or relative path=path "Build Options/Build Options.ini" ("path")) -> (appended path=w736:path)
        n328 = call <vilib>:"Check if File or Folder Exists.vi"("error in (no error)"=w731, "path"=w736) -> ("error out"=w732:errorcluster, "file or folder exists?"=w737:bool, "dup path"=w735:path)  [unwired: 7 in]
        n329 = call <vilib>:"Is Path and Not Empty.vi"("path"=w735) -> ("Is Path and Not Empty?"=w738:bool)  [unwired: 4 in]
        n330 = And(x=w738, y=w737) -> (x .and. y?=w734:bool)
        n331 = case shown="True" w734 {
          tunnel: [w758 w759] -> w747
          tunnel: w735 -> [w755 w765]
          tunnel: w730 -> [w753 w763]
          tunnel: [w753 w762] -> w733
          tunnel: w732 -> [w752 w760]
          frame False {
            n332 = Format Into String(format string="Build Options file was not found at %s.\nPlease create the build options file." ("error message (\"\")"), w755) -> (resulting string=w754:string)  [unwired: 2 in, 1 out]
            n333 = call <vilib>:"Error Cluster From Error Code.vi"("show call chain? (False)"=TRUE, "error in (no error)"=w752, "error message (\"\")"=w754, "error code (0)"=5002) -> ("error out"=w758:errorcluster)  [unwired: 5 in]
          }
          frame True {
            n334 = Open/Create/Replace File(file path (use dialog)=w765, error in=w760, access (0:read/write)=enum16{"read/write", "read-only", "write-only"}."read-only") -> (refnum out=w766:refnum<file>, error out=w768:errorcluster)  [unwired: 3 in, 1 out]
            n335 = Read from Text File(file (use dialog)=w766, error in=w768) -> (refnum out=w767:refnum<file>, text=w764:string, error out=w770:errorcluster)  [unwired: 2 in, 1 out]
            n336 = Close File(refnum=w767, error in=w770) -> (error out=w761:errorcluster)  [unwired: 1 out]
            n337 = case shown="Default" w764 {
              selector: w764 -> [_ w798]
              tunnel: [w772 w797] -> w762
              tunnel: [w771 w796] -> w759
              tunnel: w763 -> [w772 w795]
              tunnel: w761 -> [w771 w794]
              frame "" {
              }
              frame Default {
                n338 = call <vilib>:"Parse JSON.vi"("error in (no error)"=w794, "JSON String"=w798) -> ("error out"=w789:errorcluster, "JSON Tree"=w792:variant)  [unwired: 6 in, 2 out]
                n339 = call-poly <vilib>:"Get Object Parameter.vi"("error in (no error)"=w789, "Parameter Name"="Build Options", "JSON Tree In (JSON Object)"=w792) -> ("error out"=w788:errorcluster, "JSON Object"=w791:variant, "JSON Tree Out Passthrough"=w786:variant)  [unwired: 5 in, 1 out]
                n340 = Current VI's Path() -> (path=w783:path)
                n341 = call-poly <vilib>:"Get Object Parameter.vi"("error in (no error)"=w788, "Parameter Name"="Broadcast Server Port", "JSON Tree In (JSON Object)"=w791) -> ("error out"=w787:errorcluster, "Double Value"=w774:dbl)  [unwired: 5 in, 2 out]
                n342 = Build Path(base path=w783, name or relative path=path "../BroadCast Server.vi" ("path")) -> (appended path=w781:path)
                n343 = Open VI Reference(type specifier VI Refnum (for type only)=refnum<vi> refnum, vi path=w781, options=128, error in (no error)=w787) -> (vi reference=w784:refnum<vi>, error out=w777:errorcluster)  [unwired: 2 in]
                n344 = TCP Create Listener(8:w777, 9:2000 ("timeout ms (25000)"), 10:w774) -> (0:w776:errorcluster, 3:w773:refnum<k5>)  [unwired: 2 in, 1 out]
                n345 = Bundle By Name(cluster=w795, "Broadcast Server Id"=w773, "Build Options i3JSON Tree"=w786) -> (w797:T7)
                n346 = call-by-ref "Start Asynchronous Call"(reference=w784, error in=w776, "Information Package"=w798, "TCP Server"=w773) -> (reference out=w780:refnum<vi>, error out=w779:errorcluster)  [unwired: 14 in]
                n347 = Close Reference(reference=w780, error in (no error)=w779) -> (error out=w796:errorcluster)
              }
            }
          }
        }
        n348 = call-poly "Enqueue Message.vi"("Priority Message? Array"=bool[] [TRUE], "error in (no error)"=w747, "Message Array"=string[] ["Initialize SCC", "Initialize Data"], "Message Queue"=w748) -> ("error out"=w746:errorcluster)  [unwired: 6 in, 1 out]
      }
      frame "Initialize Data" {
        # "Initialize Data - Initialize the state data cluster."
        n349 = Unbundle By Name(w826) -> ("Build Options i3JSON Tree"=w810:variant)
        n350 = call-poly <vilib>:"Get Object Parameter.vi"("Parameter Name"="G3_Build_Options", "JSON Tree In (JSON Object)"=w810) -> ("error out"=w814:errorcluster, "JSON Object"=w817:variant)  [unwired: 6 in, 2 out]
        n351 = call-poly <vilib>:"Get Object Parameter.vi"("error in (no error)"=w814, "Parameter Name"="Component Locations (Recursive Search)", "JSON Tree In (JSON Object)"=w817) -> ("error out"=w813:errorcluster, "JSON Array"=w816:variant, "JSON Tree Out Passthrough"=w808:variant)  [unwired: 5 in, 1 out]
        n352 = call <vilib>:"JSON Array Size.vi"("error in (no error)"=w813, "JSON Tree In (JSON Array)"=w816) -> ("error out"=w803:errorcluster, "Array Size"=w815:i32, "JSON Tree Passthrough (JSON Array)"=w811:variant)  [unwired: 7 in]
        n353 = call-poly <vilib>:"Get Object Parameter.vi"("error in (no error)"=w803, "Parameter Name"="Snapshot Depot Directories", "JSON Tree In (JSON Object)"=w808) -> ("error out"=w804:errorcluster, "JSON Array"=w809:variant)  [unwired: 5 in, 2 out]
        n354 = call <vilib>:"JSON Array Size.vi"("error in (no error)"=w804, "JSON Tree In (JSON Array)"=w809) -> ("error out"=w802:errorcluster, "Array Size"=w805:i32, "JSON Tree Passthrough (JSON Array)"=w806:variant)  [unwired: 7 in]
        n355 = for {
          N: w815 -> [_]
          tunnel: w811 -> [w848]
          tunnel: [w844] -> w818 mode=indexing
          shift-right: [w842] -> w812
          shift-left: w803 -> [w843]
          i -> [w847]
          n356 = call-poly <vilib>:"Get Array Value at Index.vi"("error in (no error)"=w843, "Index"=w847, "JSON Tree In (JSON Array)"=w848) -> ("error out"=w842:errorcluster, "String Value"=w846:string)  [unwired: 5 in, 2 out]
          n357 = String To Path(string=w846) -> (path=w845:path)
          n358 = call "Resolve Symbolic Path.vi"("Path In"=w845) -> ("Path Out"=w844:path)  [unwired: 9 in, 1 out]
        }
        n359 = for {
          N: w805 -> [_]
          tunnel: w806 -> [w841]
          tunnel: [w837] -> w799 mode=indexing
          shift-right: [w838] -> w800
          shift-left: w802 -> [w839]
          i -> [w840]
          n360 = call-poly <vilib>:"Get Array Value at Index.vi"("error in (no error)"=w839, "Index"=w840, "JSON Tree In (JSON Array)"=w841) -> ("error out"=w838:errorcluster, "String Value"=w837:string)  [unwired: 5 in, 2 out]
        }
        n361 = Merge Errors(w800, w812) -> (w801:errorcluster)
        n362 = call-poly "Enqueue Message.vi"("error in (no error)"=w801, "Message"="Analysis Begin", "Message Queue"=w833) -> ("error out"=w831:errorcluster, "dup Message Queue"=w829:refnum<queue>)  [unwired: 7 in]
        n363 = for {
          tunnel: w818 -> [w853] mode=indexing
          tunnel: [w857] -> w825 mode=concatenating
          tunnel: "Component Definition.ini" ("pattern") -> [w856]
          tunnel: [w854] -> w824
          tunnel: w831 -> [w855]
          stop <- w854 stop-if-true
          n364 = call <vilib>:"Recursive File List.vi"("pattern"=w856, "error in (no error)"=w855, "Folder Path"=w853) -> ("error out"=w854:errorcluster, "All Files in Dir"=w857:path[])  [unwired: 4 in, 3 out]
        }
        n365 = for {
          tunnel: w825 -> [w851] mode=indexing
          tunnel: [w850] -> w821 mode=indexing
          tunnel: [w849] -> w823
          stop <- w849 stop-if-true
          n366 = call <userlib>:"Construct.vi"("Component Config File"=w851) -> ("Component"=w852:refnum<class "Component.lvclass">)  [unwired: 14 in]
          n367 = property class="Component"(reference=w852) -> (reference out=w850:refnum<class "Component.lvclass">, "Accessors:Component Operations Errors"=w849:errorcluster)  [unwired: 1 in, 1 out]
        }
        n368 = Merge Errors(w824, w823) -> (w822:errorcluster)
        n369 = call <userlib>:"Construct.vi"("Components"=w821, "error in (no error)"=w822) -> ("Build Analyzer"=w827:refnum<class "Build Analyzer.lvclass">, "error out"=w834:errorcluster)  [unwired: 12 in]
        n370 = Bundle By Name(cluster=w826, "Snapshot Depot Directories"=w799, "Components"=w821, "Build Analyzer"=w827) -> (w836:T7)
        n371 = call-poly "Enqueue Message.vi"("error in (no error)"=w834, "Message Data"=w827, "Message"="Analysis Complete", "Message Queue"=w829) -> ("error out"=w830:errorcluster)  [unwired: 6 in, 1 out]
      }
      frame "Initialize SCC" {
        n372 = Unbundle By Name(w870) -> ("Build Options i3JSON Tree"=w866:variant)
        n373 = call-poly <vilib>:"Get Object Parameter.vi"("error in (no error)"=w862, "Parameter Name"="G3_Build_Options", "JSON Tree In (JSON Object)"=w866) -> ("error out"=w861:errorcluster, "JSON Object"=w858:variant)  [unwired: 5 in, 2 out]
        n374 = call-poly <vilib>:"Get Object Parameter.vi"("error in (no error)"=w861, "Parameter Name"="SCC Config File", "JSON Tree In (JSON Object)"=w858) -> ("error out"=w860:errorcluster, "String Value"=w863:string)  [unwired: 5 in, 2 out]
        n375 = String To Path(string=w863) -> (path=w859:path)
        n376 = call "Resolve Symbolic Path.vi"("Path In"=w859) -> ("Path Out"=w867:path)  [unwired: 9 in, 1 out]
        n377 = call <userlib>:"Construct.vi"("SCC Config File"=w867, "error in (no error)"=w860) -> ("Source Code Control out"=w868:refnum<class "Abstract SCC API.lvclass">, "error out"=w869:errorcluster)  [unwired: 12 in]
        n378 = Bundle By Name(cluster=w870, "SCC Session"=w868) -> (w871:T7)
      }
      frame "Update Sync Action" {
        n379 = Unbundle By Name(w875) -> ("Sync Action"=w874:enum16{"No Sync", "Sync", "Force Sync"})
        n380 = Variant To Data(error in=w878, type=w874, Variant=w876) -> (data=w872:enum16{"No Sync", "Sync", "Force Sync"}, error out=w877:errorcluster)
        n381 = Bundle By Name(cluster=w875, "Sync Action"=w872) -> (w873:T7)
      }
      frame "Flush Ordered Exports" {
        n382 = Bundle By Name(cluster=w881, "Ordered Exports"=refnum<class "Export.lvclass">[] []) -> (w879:T7)
      }
      frame "Error" {
        # "Error - Check the error message data and respond accordingly. This message is sent by the \"Error Handler\" VIs at the end of each loop in this application."
        n383 = Variant To Data(error in=w894, type=errorcluster {"status"=FALSE, "code"=0, "source"=""} ("error constant"), Variant=w892) -> (data=w890:errorcluster, error out=w889:errorcluster)
        n384 = call <vilib>:"Simple Error Handler.vi"("error source (\" \")"="Build Engine" ("error source (\" \")"), "error in (no error)"=w890) -> ()  [unwired: 3 in, 5 out]
        n385 = call-poly "Enqueue Message.vi"("Priority Message? (F)"=TRUE, "Message"="Exit", "Message Queue"=w884) -> ("error out"=w888:errorcluster)  [unwired: 7 in, 1 out]
        n386 = Merge Errors(w888, w889) -> (w887:errorcluster)
      }
      frame "-----Build-----" {
        # "Duplicate this frame when creating new messages.  Change this comment in the duplicated frame to describe this message."
        n387 = Merge Errors(w897) -> (w895:errorcluster)
      }
      frame "Pre Build Check" {
        n388 = Variant To Data(type=refnum<class "Export.lvclass">[] [] ("Ordered Exports"), Variant=w899) -> (data=w898:refnum<class "Export.lvclass">[])  [unwired: 1 in, 1 out]
        n389 = Unbundle By Name(w903) -> ("SCC Session"=w906:refnum<class "Abstract SCC API.lvclass">)
        n390 = for {
          tunnel: w898 -> [w931] mode=indexing
          tunnel: [w929] -> w908 mode=indexing if=w928
          # "Run Commit Checks per export. Return any errors."
          n391 = property class="Export"(reference=w931) -> (reference out=w930:refnum<class "Export.lvclass">, "Accessors:Commit behavior"=w925:refnum<class "Commit.lvclass">)  [unwired: 1 in, 1 out]
          n392 = call-dynamic "Test Submit.vi"("Export in"=w930) -> ("Export out"=w926:refnum<class "Export.lvclass">, "Read for Submit"=w927:bool)  [unwired: 13 in]
          n393 = case shown="False" w927 {
            tunnel: w926 -> [w940 _]
            tunnel: [w935 _] -> w929
            tunnel: [TRUE _] -> w928
            tunnel: w925 -> [w933 _]
            frame False {
              n394 = call <vilib>:"Get LV Class Path.vi"("object"=w933) -> ("class path"=w932:path)  [unwired: 9 in, 1 out]
              n395 = call "Read Export Operation Errors.vi"("Export in"=w940) -> ("Export Operation Errors"=w938:errorcluster)  [unwired: 8 in, 2 out]
              n396 = Unbundle By Name(w938) -> ("code"=w937:i32, "source"=w936:string)
              n397 = Format Into String(format string="Commit Behavior: %s\nError Code: %d\nMessage: %s", w932, w937, w936) -> (resulting string=w935:string)  [unwired: 2 in, 1 out]
            }
            frame True {
            }
          }
        }
        n398 = call-dynamic "Initialize.vi"("SCC in"=w906) -> ("SCC out"=w901:refnum<class "Abstract SCC API.lvclass">, "Initialized"=w905:bool, "error out"=w902:errorcluster)  [unwired: 12 in]
        n399 = Bundle By Name(cluster=w903, "SCC Session"=w901, "Ordered Exports"=w898) -> (w904:T7)
        n400 = Empty Array?(array=w908) -> (empty?=w910:bool)
        n401 = And(x=w905, y=w910) -> (x .and. y?=w907:bool)
        n402 = case shown="False" w907 {
          tunnel: [w912 w923] -> w911
          tunnel: w902 -> [w915 _]
          tunnel: w908 -> [w914 _]
          tunnel: w909 -> [w913 w922]
          frame False {
            n403 = Unbundle By Name(w915) -> ("source"=w920:string)
            n404 = Build Array (concatenate)(w920, w914) -> (w921:string[])
            n405 = Array To Spreadsheet String(delimiter (Tab)="\n", array=w921, 3:"" ("format string")) -> (spreadsheet string=w919:string)
            n406 = call-poly "Enqueue Message.vi"("Message Data"=w919, "Message"="Pre Build Commit Readiness Failure", "Message Queue"=w913) -> ("error out"=w912:errorcluster)  [unwired: 7 in, 1 out]
          }
          frame True {
            n407 = call-poly "Enqueue Message.vi"("Message"="Advance Phase", "Message Queue"=w922) -> ("error out"=w923:errorcluster)  [unwired: 8 in, 1 out]
          }
        }
      }
      frame "Init Build" {
        w946 = 10  # Number of Build Groups to Keep
        n408 = Unbundle By Name(w943) -> ("Ordered Exports"=w942:refnum<class "Export.lvclass">[])
        n409 = for {
          tunnel: w942 -> [w973] mode=indexing
          # "Clean old bulds"
          n410 = call "Clear Merged Errors.vi"("Export in"=w973) -> ("Export out"=w972:refnum<class "Export.lvclass">)  [unwired: 12 in, 2 out]
          n411 = call-dynamic "Clean.vi"("Export in"=w972) -> ()  [unwired: 14 in, 1 out]
        }
        n412 = Temporary Directory() -> (w956:path)
        n413 = Get Date/Time In Seconds() -> (seconds since 1Jan1904=w954:timestamp)
        n414 = call-poly "Enqueue Message.vi"("Message"="Pre Build", "Message Queue"=w960) -> ("error out"=w959:errorcluster)  [unwired: 8 in, 1 out]
        n415 = Build Path(base path=w956, name or relative path=path "G3Build/Build_Groups" ("path")) -> (appended path=w951:path)
        n416 = Format Date/Time String(time format string (%c)="G3_Export_Group_%Y_%m_%d_%H_%M_%S", seconds (now)=w954) -> (date/time string=w953:string)  [unwired: 1 in]
        n417 = List Folder(path=w951) -> (path out=w950:path, folder names=w948:string[])  [unwired: 3 in, 2 out]
        n418 = Build Path(base path=w951, name or relative path=w953) -> (appended path=w952:path)
        n419 = Array Size(array=w948) -> (size(s)=w947:i32)
        n420 = Greater?(x=w947, y=w946) -> (0:w945:bool)
        n421 = case shown="True" w945 {
          tunnel: w948 -> [_ w967]
          tunnel: w946 -> [_ w965]
          tunnel: w950 -> [_ w964]
          frame False {
          }
          frame True {
            n422 = Sort 1D Array(array=w967) -> (sorted array=w966:string[])
            n423 = Delete From Array(array=w966, length=w965) -> (array with subset deleted=w963:string[])  [unwired: 1 in, 1 out]
            n424 = for {
              tunnel: w963 -> [w971] mode=indexing
              tunnel: w964 -> [w970]
              # "Delete all but last 10 build groups"
              n425 = Build Path(base path=w970, name or relative path=w971) -> (appended path=w969:path)
              n426 = call <userlib>:"Delete Recursive__ogtk.vi"("Recursive? (FALSE)"=TRUE, "Path"=w969) -> ()  [unwired: 8 in, 2 out]
            }
          }
        }
        n427 = call <userlib>:"Create Dir if Non-Existant__ogtk.vi"("Directory Path"=w952) -> ("error out"=→"error out":errorcluster, "dup Directory Path"=w944:path)  [unwired: 8 in, 1 out]
        n428 = Bundle By Name(cluster=w943, "Build Groups Folder"=w944, "Build Marker"=u32 0, "SCC Synchronized Paths"=variant) -> (w962:T7)
      }
      frame "Pre Build" {
        n429 = call-poly "Enqueue Message.vi"("Message"="Build", "Message Queue"=w980) -> ("error out"=w976:errorcluster)  [unwired: 8 in, 1 out]
        n430 = Unbundle By Name(w979) -> ("Build Marker"=w975:u32)
        n431 = call-poly "Enqueue Message.vi"("error in (no error)"=w976, "Message Data"=w975, "Message"="Update Build Marker", "Message Queue"=w977) -> ("error out"=w974:errorcluster)  [unwired: 6 in, 1 out]
      }
      frame "Build" {
        n432 = Unbundle By Name(w994) -> ("SCC Session"=w988:refnum<class "Abstract SCC API.lvclass">, "Ordered Exports"=w990:refnum<class "Export.lvclass">[], "Build Marker"=w991:u32, "Sync Action"=w984:enum16{"No Sync", "Sync", "Force Sync"}, "SCC Synchronized Paths"=w983:variant)
        n433 = in-place {
          in-place-border: w988 -> [w1003]
          in-place-border: [w1002] -> w985
          in-place-border: w984 -> [w1001]
          in-place-border: w983 -> [w996]
          in-place-border: [w995] -> w982
          n434 = in-place-array #1(w990, w991) -> (w1005:refnum<class "Export.lvclass">)
          n435 = case shown="\"Sync\", \"Force Sync\"" w1001 {
            selector: w1001 -> [_ w1016]
            tunnel: w1005 -> [w1009 w1021]
            tunnel: [w1009 w1020] -> w1004
            tunnel: w1003 -> [w1008 w1019]
            tunnel: [w1008 w1018] -> w1002
            tunnel: [_ w1015] -> w999
            tunnel: w996 -> [w1007 w1014]
            tunnel: [w1007 w1010] -> w995
            frame "No Sync", Default {
            }
            frame "Sync", "Force Sync" {
              n436 = property class="Export"(reference=w1021) -> (reference out=w1020:refnum<class "Export.lvclass">, "Accessors:Component Root path"=w1017:path)  [unwired: 1 in, 1 out]
              n437 = Path To String(path=w1017) -> (string=w1013:string)
              n438 = Get Variant Attribute(Variant=w1014, name=w1013) -> (duplicate Variant=w1011:variant, found=w1012:bool)  [unwired: 2 in, 2 out]
              n439 = case shown="False" w1012 {
                tunnel: w1019 -> [w1029 w1038]
                tunnel: [w1028 w1038] -> w1018
                tunnel: w1016 -> [w1022 _]
                tunnel: [w1023 _] -> w1015
                tunnel: w1013 -> [w1026 _]
                tunnel: w1011 -> [w1027 w1037]
                tunnel: [w1025 w1037] -> w1010
                frame False {
                  n440 = call-dynamic "Sync.vi"("CL_G3_VIComponentBuilder.lvlib:SCC"=w1029, "Sync Mode"=w1022, "Depot \\ Local Location"=w1026) -> ("CL_G3_VIComponentBuilder.lvlib:SCC"=w1028:refnum<class "Abstract SCC API.lvclass">, "error out"=w1024:errorcluster)  [unwired: 11 in]
                  n441 = case shown="\"Sync\", \"Force Sync\"" w1022 {
                    tunnel: w1027 -> [w1031 w1036]
                    tunnel: w1026 -> [_ w1035]
                    tunnel: [w1031 w1034] -> w1025
                    tunnel: w1024 -> [w1030 w1033]
                    tunnel: [w1030 w1032] -> w1023
                    frame "No Sync", Default {
                    }
                    frame "Sync", "Force Sync" {
                      n442 = Set Variant Attribute(Variant=w1036, name=w1035, value=w1035, error in=w1033) -> (Variant out=w1034:variant, error out=w1032:errorcluster)  [unwired: 1 out]
                    }
                  }
                }
                frame True {
                }
              }
            }
          }
          n443 = property class="Export"(reference=w1004, "Accessors:Merged Errors"=w999) -> (reference out=w1000:refnum<class "Export.lvclass">)  [unwired: 1 in, 1 out]
          n444 = call-dynamic "Pre Build.vi"("Export In"=w1000) -> ("Export out"=w998:refnum<class "Export.lvclass">)  [unwired: 14 in]
          n445 = call-dynamic "Build.vi"("Export In"=w998) -> ("Export Out"=w997:refnum<class "Export.lvclass">)  [unwired: 14 in]
          n446 = call-dynamic "Post Build.vi"("Export In"=w997) -> ("Export out"=w1006:refnum<class "Export.lvclass">)  [unwired: 14 in]
          n447 = in-place-array #1(w1006) -> (w989:refnum<class "Export.lvclass">[])  [unwired: 1 out]
        }
        n448 = call-poly "Enqueue Message.vi"("Message"="Post Build", "Message Queue"=w992) -> ("error out"=w986:errorcluster)  [unwired: 8 in, 1 out]
        n449 = Bundle By Name(cluster=w994, "SCC Session"=w985, "Ordered Exports"=w989, "SCC Synchronized Paths"=w982) -> (w993:T7)
      }
      frame "Post Build" {
        w1051 = T15 {"Ordered Exports"=[], "Build Marker"=0, "Build Groups Folder"=path "", "Build Engine Queue"=refnum, "error out"={"status"=FALSE, "code"=0, "source"=""}}  # Sequence Locals
        w1049 = string[] ["Report Final Build Status", "Write to Group Export Mainfest", "Copy Export to Group Export Folder", "Enqueue Command to Build Engine"]  # Sequences
        n450 = Unbundle By Name(w1046) -> ("Ordered Exports"=w1043:refnum<class "Export.lvclass">[], "Build Marker"=w1042:u32, "Build Groups Folder"=w1041:path)
        n451 = Bundle By Name(cluster=w1051, "Ordered Exports"=w1043, "Build Marker"=w1042, "Build Groups Folder"=w1041, "Build Engine Queue"=w1047) -> (w1048:T15)
        n452 = for {
          tunnel: w1049 -> [w1053] mode=indexing
          shift-right: [w1054] -> w1050
          shift-left: w1048 -> [w1055]
          tunnel: w1040 -> [w1052]
          n453 = case shown="\"Enqueue Command to Build Engine\"" w1053 {
            selector: w1053 -> [w1059 _ _ _ _]
            tunnel: w1055 -> [w1062 w1069 w1098 w1117 w1130]
            tunnel: [w1057 w1069 w1073 w1111 w1129] -> w1054
            tunnel: w1052 -> [_ w1064 _ _ _]
            frame "Bad Command", Default {
              n454 = Format Into String(format string="Sequence \"%s\" has no case designed to handle it.", w1059) -> (resulting string=w1058:string)  [unwired: 2 in, 1 out]
              n455 = Bundle By Name(cluster=errorcluster {"status"=TRUE, "code"=9999, "source"=""} ("error out"), "source"=w1058) -> (w1056:errorcluster)
              n456 = Bundle By Name(cluster=w1062, "error out"=w1056) -> (w1057:T15)
            }
            frame "Report Final Build Status" {
              n457 = Unbundle By Name(w1069) -> ("Ordered Exports"=w1068:refnum<class "Export.lvclass">[], "Build Marker"=w1067:u32)
              n458 = Index Array(array=w1068, index=w1067) -> (element=w1066:refnum<class "Export.lvclass">)
              n459 = property class="Export"(reference=w1066) -> ("Accessors:Merged Errors"=w1063:errorcluster)  [unwired: 1 in, 2 out]
              n460 = call-poly "Enqueue Message.vi"("Message Data"=w1063, "Message"="Final Build Status", "Message Queue"=w1064) -> ()  [unwired: 7 in, 2 out]
            }
            frame "Write to Group Export Mainfest" {
              w1081 = T16 {"Export Path"=path "", "Export Files"=[]}  # Exports
              n461 = Unbundle By Name(w1098) -> ("Build Groups Folder"=w1093:path, "Ordered Exports"=w1092:refnum<class "Export.lvclass">[], "Build Marker"=w1091:u32)
              n462 = Index Array(array=w1092, index=w1091) -> (element=w1090:refnum<class "Export.lvclass">)
              n463 = Strip Path(path=w1093) -> (name=w1096:string)  [unwired: 1 out]
              n464 = property class="Export"(reference=w1090) -> ("Accessors:Component Export Directory"=w1089:path, "Accessors:Product Name"=w1074:string)  [unwired: 1 in, 2 out]
              n465 = Format Into String(format string="%s.ini", w1096) -> (resulting string=w1095:string)  [unwired: 2 in, 1 out]
              n466 = Build Path(base path=w1093, name or relative path=w1095) -> (appended path=w1094:path)
              n467 = call <vilib>:"Open Config Data.vi"("configuration file path"=w1094) -> ("error out"=w1077:errorcluster, "refnum"=w1083:T17)  [unwired: 8 in, 1 out]
              n468 = call <vilib>:"Get Section Names.vi"("error in (no error)"=w1077, "refnum"=w1083) -> ("error out"=w1076:errorcluster, "section names"=w1080:string[], "refnum out"=w1082:T17)  [unwired: 7 in]
              n469 = for {
                shift-right: [w1102] -> w1079
                shift-left: w1082 -> [w1105]
                tunnel: w1081 -> [w1104]
                tunnel: w1080 -> [w1106] mode=indexing
                tunnel: [w1101] -> w1078 mode=concatenating
                shift-right: [w1099] -> w1072
                shift-left: w1076 -> [w1100]
                n470 = call <userlib>:"Read Section Cluster__ogtk.vi"("section (optional)"=w1106, "error in (no error)"=w1100, "Section Formatted Cluster Type"=w1104, "refnum"=w1105) -> ("error out"=w1107:errorcluster, "Section Formatted Cluster"=w1108:variant, "dup refnum"=w1102:T17)  [unwired: 3 in, 2 out]
                n471 = Variant To Data(error in=w1107, type=w1104, Variant=w1108) -> (data=w1103:T16, error out=w1099:errorcluster)
                n472 = Unbundle By Name(w1103) -> ("Export Files"=w1101:string[])
              }
              n473 = List Folder(path=w1089, error in=w1072) -> (path out=w1075:path, filenames=w1085:string[], error out=w1071:errorcluster)  [unwired: 2 in, 1 out]
              n474 = call-poly <userlib>:"Filter 1D Array__ogtk.vi"("items to filter"=w1078, "array"=w1085) -> ("filtered array"=w1084:string[])  [unwired: 4 in, 1 out]
              n475 = Bundle By Name(cluster=w1081, "Export Files"=w1084, "Export Path"=w1075) -> (w1087:T16)
              n476 = call <userlib>:"Write Section Cluster__ogtk.vi"("section (optional)"=w1074, "error in (no error)"=w1071, "Section Formatted Cluster"=w1087, "refnum"=w1079) -> ("error out"=w1086:errorcluster, "dup refnum"=w1088:T17)  [unwired: 6 in]
              n477 = call <vilib>:"Close Config Data.vi"("error in (no error)"=w1086, "refnum"=w1088) -> ("error out"=w1070:errorcluster)  [unwired: 8 in, 1 out]
              n478 = Bundle By Name(cluster=w1098, "error out"=w1070) -> (w1073:T15)
            }
            frame "Copy Export to Group Export Folder" {
              n479 = Unbundle By Name(w1117) -> ("Ordered Exports"=w1116:refnum<class "Export.lvclass">[], "Build Marker"=w1115:u32, "Build Groups Folder"=w1109:path)
              n480 = Index Array(array=w1116, index=w1115) -> (element=w1114:refnum<class "Export.lvclass">)
              n481 = property class="Export"(reference=w1114) -> (error out=w1113:errorcluster, "Accessors:Component Export Directory"=w1120:path)  [unwired: 1 in, 1 out]
              n482 = List Folder(path=w1120, error in=w1113) -> (path out=w1119:path, filenames=w1118:string[], error out=w1112:errorcluster)  [unwired: 2 in, 1 out]
              n483 = for {
                tunnel: w1109 -> [w1127]
                tunnel: w1119 -> [w1126]
                tunnel: w1118 -> [w1125] mode=indexing
                shift-right: [w1121] -> w1110
                shift-left: w1112 -> [w1122]
                n484 = Build Path(base path=w1126, name or relative path=w1125) -> (appended path=w1124:path)
                n485 = Copy(8:w1122, 9:TRUE ("overwrite (F)"), 10:w1127, 11:w1124) -> (0:w1121:errorcluster)  [unwired: 1 in, 2 out]
              }
              n486 = Bundle By Name(cluster=w1117, "error out"=w1110) -> (w1111:T15)
            }
            frame "Enqueue Command to Build Engine" {
              n487 = Unbundle By Name(w1130) -> ("Build Marker"=w1135:u32, "Ordered Exports"=w1136:refnum<class "Export.lvclass">[], "Build Engine Queue"=w1128:refnum<queue>)
              n488 = Array Size(array=w1136) -> (size(s)=w1132:i32)
              n489 = Decrement(x=w1132) -> (x-1=w1133:i32)
              n490 = Greater Or Equal?(x=w1135, y=w1133) -> (x >= y?=w1134:bool)
              n491 = case shown="False" w1134 {
                tunnel: w1130 -> [w1141 w1142]
                tunnel: [w1140 w1142] -> w1129
                tunnel: ["Pre Build" ("f") "Build Complete" ("f")] -> w1131
                tunnel: w1135 -> [w1138 _]
                frame False {
                  n492 = Increment(x=w1138) -> (x+1=w1137:u32)
                  n493 = Bundle By Name(cluster=w1141, "Build Marker"=w1137) -> (w1140:T15)
                }
                frame True {
                }
              }
              n494 = call-poly "Enqueue Message.vi"("Message"=w1131, "Message Queue"=w1128) -> ()  [unwired: 8 in, 2 out]
            }
          }
        }
        n495 = Unbundle By Name(w1050) -> ("Build Marker"=w1044:u32, "error out"=w1039:errorcluster)
        n496 = Bundle By Name(cluster=w1046, "Build Marker"=w1044) -> (w1045:T7)
      }
      frame "Build Complete" {
        n497 = Unbundle By Name(w1148) -> ("Build Groups Folder"=w1145:path, "Ordered Exports"=w1144:refnum<class "Export.lvclass">[])
        n498 = Bundle By Name(cluster=T13 {"Ordered Exports"=[], "Build Groups Folder"=path ""} ("input cluster"), "Build Groups Folder"=w1145, "Ordered Exports"=w1144) -> (w1146:T13)
        n499 = call-poly "Enqueue Message.vi"("Message Data"=w1146, "Message"="Advance Phase", "Message Queue"=w1150) -> ()  [unwired: 7 in, 2 out]
      }
      frame "Abort" {
        n500 = Unbundle By Name(w1159) -> ("Ordered Exports"=w1156:refnum<class "Export.lvclass">[], "Build Marker"=w1158:u32)
        n501 = Flush Queue(queue=w1153) -> (queue out=w1152:refnum<queue>)  [unwired: 1 in, 2 out]
        n502 = Increment(x=w1158) -> (x+1=w1154:u32)
        n503 = call-poly "Enqueue Message.vi"("Message"="Build Complete", "Message Queue"=w1152) -> ()  [unwired: 8 in, 2 out]
        n504 = Split 1D Array(array=w1156, index=w1154) -> (first subarray=w1155:refnum<class "Export.lvclass">[])  [unwired: 1 out]
        n505 = Bundle By Name(cluster=w1159, "Ordered Exports"=w1155) -> (w1157:T7)
      }
      frame "Build Submission Recipe" {
        # "#ToDo: Build up a recipie for submission\nand use that in case submission fails half\nway through."
        n506 = call-poly "Enqueue Message.vi"("Message"="Execute Commit", "Message Queue"=w1163) -> ()  [unwired: 8 in, 2 out]
      }
      frame "---Commit---" {
      }
      frame "Pre Execute Commit" {
        n507 = disable-structure shown="Enabled" {
          disable-tunnel: w1173 -> [w1179 _]
          disable-tunnel: [w1177 _] -> w1169
          disable-tunnel: [w1175 TRUE ("empty?")] -> w1168
          frame Disabled {
            n508 = Unbundle By Name(w1179) -> ("Ordered Exports"=w1176:refnum<class "Export.lvclass">[])
            n509 = for {
              tunnel: w1176 -> [w1188] mode=indexing
              shift-right: [w1186] -> _
              shift-left: variant -> [w1185]
              tunnel: [w1181] -> w1177 mode=indexing if=w1180
              # "Run Commit Checks. Return any errors."
              n510 = property class="Export"(reference=w1188) -> (reference out=w1184:refnum<class "Export.lvclass">, "Accessors:Commit behavior"=w1187:refnum<class "Commit.lvclass">)  [unwired: 1 in, 1 out]
              n511 = call <vilib>:"Get LV Class Name.vi"("object"=w1187) -> ("class name"=w1182:string)  [unwired: 9 in, 1 out]
              n512 = Set Variant Attribute(Variant=w1185, name=w1182, value=w1182) -> (Variant out=w1186:variant, replaced=w1183:bool)  [unwired: 1 in, 1 out]
              n513 = case shown="False" w1183 {
                tunnel: w1184 -> [w1194 _]
                tunnel: [w1189 _] -> w1180
                tunnel: w1182 -> [w1191 _]
                tunnel: [w1190 _] -> w1181
                frame False {
                  n514 = call-dynamic "Test Submit.vi"("Export in"=w1194) -> ("Export out"=w1192:refnum<class "Export.lvclass">, "Read for Submit"=w1193:bool)  [unwired: 13 in]
                  n515 = case shown="False" w1193 {
                    tunnel: w1192 -> [w1202 _]
                    tunnel: w1191 -> [w1197 _]
                    tunnel: [w1196 _] -> w1190
                    tunnel: [TRUE _] -> w1189
                    frame False {
                      n516 = call "Read Export Operation Errors.vi"("Export in"=w1202) -> ("Export Operation Errors"=w1200:errorcluster)  [unwired: 8 in, 2 out]
                      n517 = Unbundle By Name(w1200) -> ("code"=w1199:i32, "source"=w1198:string)
                      n518 = Format Into String(format string="Commit Behavior: %s\nError Code: %d\nMessage: %s", w1197, w1199, w1198) -> (resulting string=w1196:string)  [unwired: 2 in, 1 out]
                    }
                    frame True {
                    }
                  }
                }
                frame True {
                }
              }
            }
            n519 = Empty Array?(array=w1177) -> (empty?=w1175:bool)
          }
          frame Enabled {
            # "Commenting this out becuase we are doing prechecks pre build\nif people complain we can bring this back."
          }
        }
        n520 = case shown="True" w1168 {
          tunnel: w1173 -> [w1209 w1212]
          tunnel: [w1209 w1212] -> w1174
          tunnel: w1172 -> [w1211 _]
          tunnel: [w1208 w1215] -> w1171
          tunnel: w1170 -> [_ w1214]
          tunnel: w1169 -> [w1204 _]
          frame False {
            n521 = Array To Spreadsheet String(delimiter (Tab)="\n", array=w1204, 3:"" ("format string")) -> (spreadsheet string=w1205:string)
            n522 = call-poly "Enqueue Message.vi"("Message Data"=w1205, "Message"="Commit Readiness Failure", "Message Queue"=w1211) -> ("error out"=w1208:errorcluster)  [unwired: 7 in, 1 out]
          }
          frame True {
            n523 = call-poly "Enqueue Message.vi"("Message"="Execute Commit", "Message Queue"=w1214) -> ("error out"=w1215:errorcluster)  [unwired: 8 in, 1 out]
          }
        }
      }
      frame "Commit" {
        n524 = call-poly "Enqueue Message.vi"("Message"="Pre Execute Commit", "Message Queue"=w1218) -> ("error out"=w1216:errorcluster)  [unwired: 8 in, 1 out]
      }
      frame "Execute Commit" {
        w1233 = T18 {"SCC Session"=refnum, "Failed Submissions"=[], "All Exports"=[], "Exports W\\O Errors"=[], "Ordered Expors"=[]}  # Local Data
        w1231 = string[] ["Create New Changelist", "Add Export Artifacts to SCC and Commit", "Submit Changelist and Create P4 Labels", "Update P4 Changelist"]  # Sequences
        n525 = Unbundle By Name(w1225) -> ("Ordered Exports"=w1227:refnum<class "Export.lvclass">[], "SCC Session"=w1224:refnum<class "Abstract SCC API.lvclass">, "Snapshot Depot Directories"=w1220:string[])
        n526 = Bundle By Name(cluster=w1233, "Ordered Expors"=w1227, "SCC Session"=w1224) -> (w1230:T18)
        n527 = for {
          tunnel: w1231 -> [w1240] mode=indexing
          shift-right: [w1242] -> w1232
          shift-left: w1230 -> [w1243]
          tunnel: [w1238] -> w1226
          tunnel: w1220 -> [w1237]
          stop <- w1238 stop-if-true
          n528 = case shown="\"Add Export Artifacts to SCC and Commit\"" w1240 {
            selector: w1240 -> [w1256 _ _ _ _]
            tunnel: w1243 -> [w1261 w1264 w1276 w1314 w1336]
            tunnel: [w1261 w1263 w1274 w1313 w1335] -> w1242
            tunnel: [w1258 w1262 _ w1312 w1333] -> w1241
            tunnel: ["" ("Accessors:Name") _ _ _ _] -> w1239
            tunnel: w1237 -> [_ _ _ w1307 _]
            frame "Bad Command", Default {
              n529 = Format Into String(format string="Sequence \"%s\" has no case designed to handle it.", w1256) -> (resulting string=w1255:string)  [unwired: 2 in, 1 out]
              n530 = Bundle By Name(cluster=errorcluster {"status"=TRUE, "code"=9999, "source"=""} ("error out"), "source"=w1255) -> (w1258:errorcluster)
            }
            frame "Create New Changelist" {
              n531 = in-place {
                in-place-border: [w1265] -> w1262
                n532 = in-place-cluster #2(w1264) -> ("SCC Session"=w1268:refnum<class "Abstract SCC API.lvclass">)
                n533 = call-dynamic "Create New Changelist.vi"("SCC in"=w1268, "Changelist Description"="Auto build by svc_labview" ("Description")) -> ("SCC out"=w1267:refnum<class "Abstract SCC API.lvclass">, "error out"=w1265:errorcluster)  [unwired: 12 in]
                n534 = in-place-cluster #2("SCC Session"=w1267) -> (w1263:T18)
              }
            }
            frame "Add Export Artifacts to SCC and Commit" {
              n535 = Unbundle By Name(w1276) -> ("SCC Session"=w1269:refnum<class "Abstract SCC API.lvclass">, "Ordered Expors"=w1275:refnum<class "Export.lvclass">[])
              n536 = for {
                shift-right: [w1288] -> w1270
                shift-left: w1269 -> [w1290]
                tunnel: [w1281] -> w1273 mode=indexing
                tunnel: [w1281] -> w1271 mode=indexing if=w1287
                tunnel: [w1281] -> w1272 mode=indexing if=w1279
                tunnel: w1275 -> [w1286] mode=indexing
                # "Add Each export artifact to a change list, commit. On comitt failure remove items from change list."
                n537 = property class="Export"(reference=w1286) -> (reference out=w1284:refnum<class "Export.lvclass">, "Accessors:Export Artifacts for SCC"=w1278:path[])  [unwired: 1 in, 1 out]
                n538 = Path To String(path=w1278) -> (string=w1277:string[])
                n539 = for {
                  tunnel: w1277 -> [w1304] mode=indexing
                  shift-right: [w1305] -> w1289
                  shift-left: w1290 -> [w1306]
                  tunnel: [w1303] -> w1285
                  tunnel: [w1304] -> w1283 mode=indexing
                  stop <- w1303 stop-if-true
                  n540 = call-dynamic "Add File or Folder to Changelist.vi"("SCC in"=w1306, "File Path"=w1304) -> ("SCC out"=w1305:refnum<class "Abstract SCC API.lvclass">, "error out"=w1303:errorcluster)  [unwired: 12 in]
                }
                n541 = case shown="No Error" w1285 {
                  selector: w1285 -> [_ w1295]
                  tunnel: [w1292 w1293] -> w1282
                  tunnel: w1284 -> [w1291 w1294]
                  frame No Error {
                    n542 = call-dynamic "Submit.vi"("Export In"=w1291) -> ("Export Out"=w1292:refnum<class "Export.lvclass">)  [unwired: 14 in]
                  }
                  frame Error {
                    n543 = property class="Export"(reference=w1294, "Accessors:Merged Errors"=w1295) -> (reference out=w1293:refnum<class "Export.lvclass">)  [unwired: 1 in, 1 out]
                  }
                }
                n544 = property class="Export"(reference=w1282) -> (reference out=w1281:refnum<class "Export.lvclass">, "Accessors:Merged Errors"=w1280:errorcluster)  [unwired: 1 in, 1 out]
                n545 = Unbundle By Name(w1280) -> ("status"=w1279:bool)
                n546 = case shown="Error" w1280 {
                  tunnel: w1289 -> [w1296 w1299]
                  tunnel: [w1296 w1298] -> w1288
                  tunnel: w1283 -> [_ w1297]
                  frame No Error {
                  }
                  frame Error {
                    n547 = for {
                      shift-right: [w1301] -> w1298
                      shift-left: w1299 -> [w1302]
                      tunnel: w1297 -> [w1300] mode=indexing
                      n548 = call-dynamic "Revert File or Folder in Changelist.vi"("SCC in"=w1302, "File Path"=w1300) -> ("SCC out"=w1301:refnum<class "Abstract SCC API.lvclass">)  [unwired: 12 in, 1 out]
                    }
                  }
                }
                n549 = Not(x=w1279) -> (.not. x?=w1287:bool)
              }
              n550 = Bundle By Name(cluster=w1276, "SCC Session"=w1270, "Failed Submissions"=w1272, "Exports W\\O Errors"=w1271, "All Exports"=w1273) -> (w1274:T18)
            }
            frame "Submit Changelist and Create P4 Labels" {
              n551 = Unbundle By Name(w1314) -> ("SCC Session"=w1311:refnum<class "Abstract SCC API.lvclass">, "Exports W\\O Errors"=w1309:refnum<class "Export.lvclass">[])
              n552 = Empty Array?(array=w1309) -> (empty?=w1308:bool)
              n553 = case shown="False" w1308 {
                tunnel: [w1322 _] -> w1312
                tunnel: w1311 -> [w1317 w1332]
                tunnel: [w1320 w1332] -> w1310
                tunnel: w1309 -> [w1316 _]
                tunnel: w1307 -> [w1315 _]
                frame False {
                  n554 = call-dynamic "Submit.vi"("SCC in"=w1317) -> ("SCC out"=w1321:refnum<class "Abstract SCC API.lvclass">, "error out"=w1319:errorcluster)  [unwired: 13 in]
                  n555 = for {
                    tunnel: [w1324] -> w1318 mode=indexing
                    shift-right: [w1326] -> w1320
                    shift-left: w1321 -> [w1327]
                    tunnel: w1316 -> [w1328] mode=indexing
                    tunnel: w1315 -> [w1323]
                    # "Create P4 Label for successful submissions"
                    n556 = property class="Export"(reference=w1328) -> ("Accessors:Unique Name"=w1331:string, "Accessors:Built Version"=w1329:string)  [unwired: 1 in, 2 out]
                    n557 = Concatenate Strings(w1331, "-" ("string"), w1329) -> (w1325:string)
                    n558 = call-dynamic "Take Snapshot.vi"("SCC in"=w1327, "Label Text"=w1325, "Directories to Snapshot"=w1323) -> ("SCC out"=w1326:refnum<class "Abstract SCC API.lvclass">, "error out"=w1324:errorcluster)  [unwired: 11 in]
                  }
                  n559 = Merge Errors(w1319, w1318) -> (w1322:errorcluster)
                }
                frame True {
                }
              }
              n560 = Bundle By Name(cluster=w1314, "SCC Session"=w1310) -> (w1313:T18)
            }
            frame "Update P4 Changelist" {
              n561 = Unbundle By Name(w1336) -> ("SCC Session"=w1339:refnum<class "Abstract SCC API.lvclass">, "Exports W\\O Errors"=w1338:refnum<class "Export.lvclass">[])
              n562 = Empty Array?(array=w1338) -> (empty?=w1337:bool)
              n563 = case shown="False" w1337 {
                tunnel: [w1346 _] -> w1333
                tunnel: w1339 -> [w1351 w1359]
                tunnel: [w1348 w1359] -> w1334
                tunnel: w1338 -> [w1352 _]
                frame False {
                  w1340 = "\n" ("delimiter (Tab)")
                  n564 = for {
                    tunnel: w1352 -> [w1358] mode=indexing
                    tunnel: [w1353] -> w1344 mode=indexing
                    n565 = property class="Export"(reference=w1358) -> ("Accessors:Product Name"=w1356:string, "Accessors:Built Version"=w1355:string, "Accessors:Unique Name"=w1354:string)  [unwired: 1 in, 2 out]
                    n566 = Format Into String(format string="%s, %s, %s", w1356, w1355, w1354) -> (resulting string=w1353:string)  [unwired: 2 in, 1 out]
                  }
                  n567 = call-dynamic "Get Changelist Description.vi"("SCC in"=w1351) -> ("SCC out"=w1349:refnum<class "Abstract SCC API.lvclass">, "Changelist Description"=w1350:string, "error out"=w1347:errorcluster)  [unwired: 12 in]
                  n568 = Array To Spreadsheet String(delimiter (Tab)=w1340, array=w1344, 3:"" ("format string")) -> (spreadsheet string=w1343:string)
                  n569 = call <vilib>:"Trim Whitespace.vi"("string"=w1343) -> ("trimmed string"=w1341:string)  [unwired: 1 in]
                  n570 = Concatenate Strings(w1350, w1340, w1341) -> (w1345:string)
                  n571 = call-dynamic "Set Changelist Description.vi"("SCC in"=w1349, "Changelist Description"=w1345, "error in (no error)"=w1347) -> ("SCC out"=w1348:refnum<class "Abstract SCC API.lvclass">, "error out"=w1346:errorcluster)  [unwired: 11 in]
                }
                frame True {
                }
              }
              n572 = Bundle By Name(cluster=w1336, "SCC Session"=w1334) -> (w1335:T18)
            }
          }
          n573 = case shown="No Error" w1241 {
            selector: w1241 -> [w1244 w1247]
            tunnel: [w1244 w1252] -> w1238
            tunnel: w1240 -> [_ w1250]
            tunnel: w1239 -> [_ w1245]
            frame No Error {
            }
            frame Error {
              n574 = Unbundle By Name(w1247) -> ("source"=w1246:string)
              n575 = Format Into String(format string="Execution Failure During Sequence \"%s\".\n \nError:\n%s\n\n%s" ("error message (\"\")"), initial string="", w1250, w1246, w1245) -> (resulting string=w1251:string)  [unwired: 1 in, 1 out]
              n576 = call <vilib>:"Error Cluster From Error Code.vi"("show call chain? (False)"=TRUE, "error message (\"\")"=w1251, "error code (0)"=9999) -> ("error out"=w1252:errorcluster)  [unwired: 6 in]
            }
          }
        }
        n577 = Unbundle By Name(w1232) -> ("Failed Submissions"=w1229:refnum<class "Export.lvclass">[], "SCC Session"=w1228:refnum<class "Abstract SCC API.lvclass">, "All Exports"=w1222:refnum<class "Export.lvclass">[], "Exports W\\O Errors"=w1221:refnum<class "Export.lvclass">[])
        n578 = Bundle By Name(cluster=w1225, "Failed Submissions"=w1229, "SCC Session"=w1228, "All Attempted Submissions"=w1222, "Successful Submissions"=w1221) -> (w1236:T7)
        n579 = call-poly "Enqueue Message.vi"("error in (no error)"=w1226, "Message"="Post Commit", "Message Queue"=w1235) -> ("error out"=w1223:errorcluster)  [unwired: 7 in, 1 out]
      }
      frame "Post Commit" {
        # "#ToDo: Handle errors better"
        n580 = Unbundle By Name(w1361) -> ("Failed Submissions"=w1364:refnum<class "Export.lvclass">[], "Successful Submissions"=w1362:refnum<class "Export.lvclass">[])
        n581 = for {
          tunnel: w1362 -> [w1393] mode=indexing
          shift-right: [w1391] -> w1368
          shift-left: variant -> [w1392]
          # "Get all types of comitt behaviors"
          n582 = property class="Export"(reference=w1393) -> ("Accessors:Commit behavior"=w1390:refnum<class "Commit.lvclass">)  [unwired: 1 in, 2 out]
          n583 = property class="Commit"(reference=w1390) -> (reference out=w1388:refnum<class "Commit.lvclass">, "Accessors:Errors"=w1389:errorcluster)  [unwired: 1 in, 1 out]
          n584 = case shown="No Error" w1389 {
            tunnel: w1392 -> [w1397 w1398]
            tunnel: [w1396 w1398] -> w1391
            tunnel: w1388 -> [w1394 _]
            frame No Error {
              n585 = call <vilib>:"Get LV Class Name.vi"("object"=w1394) -> ("class name"=w1395:string)  [unwired: 9 in, 1 out]
              n586 = Set Variant Attribute(Variant=w1397, name=w1395, value=w1394) -> (Variant out=w1396:variant)  [unwired: 1 in, 2 out]
            }
            frame Error {
            }
          }
        }
        n587 = for {
          tunnel: w1364 -> [w1384] mode=indexing
          # "Clean all Exports that had errors. Return errors from cleaning."
          n588 = call "Clear Merged Errors.vi"("Export in"=w1384) -> ("Export out"=w1383:refnum<class "Export.lvclass">)  [unwired: 12 in, 2 out]
          n589 = call-dynamic "Clean.vi"("Export in"=w1383) -> ()  [unwired: 14 in, 1 out]
        }
        n590 = Get Variant Attribute(Variant=w1368) -> (values=w1367:variant[])  [unwired: 3 in, 3 out]
        n591 = Variant To Data(type=refnum<class "Commit.lvclass">[] [], Variant=w1367) -> (data=w1365:refnum<class "Commit.lvclass">[])  [unwired: 1 in, 1 out]
        n592 = for {
          tunnel: w1365 -> [w1387] mode=indexing
          tunnel: [w1385] -> w1363 mode=indexing
          # "For each commit type, run post commit. This is old CODA+"
          n593 = call-dynamic "Post Submit.vi"("Commit in"=w1387) -> ("Commit out"=w1386:refnum<class "Commit.lvclass">)  [unwired: 14 in]
          n594 = property class="Commit"(reference=w1386) -> ("Accessors:Errors"=w1385:errorcluster)  [unwired: 1 in, 2 out]
        }
        n595 = Unbundle By Name(w1361) -> ("All Attempted Submissions"=w1360:refnum<class "Export.lvclass">[])
        n596 = Bundle By Name(cluster=w1361, "Ordered Exports"=refnum<class "Export.lvclass">[] []) -> (w1371:T7)
        n597 = flat-sequence {
          tunnel: w1373 -> [w1382]
          tunnel: [w1380] -> w1372
          tunnel: w1363 -> [w1379]
          tunnel: w1360 -> [w1374]
          frame #0 {
            # "If there are any commit errors still send the commit complete command."
            n598 = call-poly "Enqueue Message.vi"("Message"="Commit Complete", "Message Queue"=w1382) -> ("error out"=w1376:errorcluster, "dup Message Queue"=w1377:refnum<queue>)  [unwired: 8 in]
            n599 = call-poly "Enqueue Message.vi"("error in (no error)"=w1376, "Message Data"=w1374, "Message"="Advance Phase", "Message Queue"=w1377) -> ("error out"=w1375:errorcluster)  [unwired: 6 in, 1 out]
            n600 = Merge Errors(w1379, w1375) -> (w1380:errorcluster)
          }
        }
      }
      frame "Clean Exports" {
        # "All Exports"
        n601 = Unbundle By Name(w1408) -> ("Ordered Exports"=w1401:refnum<class "Export.lvclass">[])
        n602 = for {
          tunnel: [w1412] -> w1400 mode=indexing
          tunnel: w1401 -> [w1410] mode=indexing
          tunnel: [w1411] -> w1399 mode=indexing
          # "Clear all previous errors in the export. Clean All Exports. If a package isn't unregistered that's an error."
          n603 = call "Clear Merged Errors.vi"("Export in"=w1410) -> ("Export out"=w1409:refnum<class "Export.lvclass">)  [unwired: 12 in, 2 out]
          n604 = call-dynamic "Clean.vi"("Export in"=w1409) -> ("Export out"=w1413:refnum<class "Export.lvclass">)  [unwired: 14 in]
          n605 = property class="Export"(reference=w1413) -> (reference out=w1412:refnum<class "Export.lvclass">, "Accessors:Merged Errors"=w1411:errorcluster)  [unwired: 1 in, 1 out]
        }
        n606 = Bundle By Name(cluster=w1408, "Ordered Exports"=refnum<class "Export.lvclass">[] []) -> (w1403:T7)
        n607 = call-poly "Enqueue Message.vi"("Message Data"=w1400, "Message"="Exports Cleaned", "Message Queue"=w1407) -> ("error out"=w1405:errorcluster)  [unwired: 7 in, 1 out]
        n608 = Merge Errors(w1399, w1405) -> (w1404:errorcluster)
      }
      frame "Exit" {
        # "Release the message queue reference"
        # "Exit - Exit the application."
        n609 = Unbundle By Name(w1424) -> ("Broadcast Server Id"=w1415:refnum<k5>, "Components"=w1416:refnum<class "Component.lvclass">[], "SCC Session"=w1420:refnum<class "Abstract SCC API.lvclass">, "Build Analyzer"=w1425:refnum<class "Build Analyzer.lvclass">, "Ordered Exports"=w1421:refnum<class "Export.lvclass">[])
        n610 = Release Queue(queue=w1428, error in (no error)=w1426) -> (error out=w1423:errorcluster)  [unwired: 1 in, 2 out]
        n611 = TCP Close Connection(connection ID=w1415) -> (error out=w1414:errorcluster)  [unwired: 2 in, 1 out]
        n612 = for {
          tunnel: w1416 -> [w1429] mode=indexing
          n613 = call "Get All Exports.vi"("Component in"=w1429) -> ("Component out"=w1431:refnum<class "Component.lvclass">, "Exports"=w1430:refnum<class "Export.lvclass">[])  [unwired: 13 in]
          n614 = for {
            shift-right: [w1434] -> w1432
            shift-left: w1431 -> [w1434]
            tunnel: w1430 -> [w1433] mode=indexing
            n615 = call-dynamic "Deconstruct.vi"("Export In"=w1433) -> ()  [unwired: 15 in]
          }
          n616 = call-dynamic "Deconstruct.vi"("Component in"=w1432) -> ()  [unwired: 15 in]
        }
        n617 = for {
          shift-right: [w1437] -> w1422
          shift-left: w1423 -> [w1437]
          tunnel: w1421 -> [w1436] mode=indexing
          n618 = call-dynamic "Clean.vi"("Export in"=w1436) -> ("Export out"=w1435:refnum<class "Export.lvclass">)  [unwired: 14 in]
          n619 = call-dynamic "Deconstruct.vi"("Export In"=w1435) -> ()  [unwired: 15 in]
        }
        n620 = call <vilib>:"Clear Errors.vi"("error in (no error)"=w1414) -> ()  [unwired: 5 in, 2 out]
        n621 = call-dynamic "Deconstruct.vi"("SCC in"=w1420) -> ("error out"=w1418:errorcluster)  [unwired: 14 in]
        n622 = call "Deconstruct.vi"("Build Analyzer"=w1425, "error in (no error)"=w1422) -> ("error out"=w1419:errorcluster)  [unwired: 13 in]
        n623 = Merge Errors(w1418, w1419) -> (w1417:errorcluster)
      }
      frame Default {
        # "'Default' case only runs if there is a message that isn't defined in any of the other cases.  Output a programming error."
        n624 = xnode "Error Ring"("parameter 0"=w1438) -> ("error out"=w1439:errorcluster)
      }
    }
    n625 = call "Error Handler - Message Handling Loop.vi"("error in (no error)"=w720, "Message Queue"=w718) -> ("dup error in"=w719:errorcluster)  [unwired: 8 in, 1 out]
  }
  n626 = while {
    tunnel: w10 -> [w1454]
    shift-right: [w1452] -> w9
    shift-left: w7 -> [w1453]
    tunnel: [w1448] -> w8
    stop <- w1450 stop-if-true
    # "Event Handling Loop"
    n627 = event shown="[11] \"Next Button\": Value Change" {
      selector: w1453 -> [_ _ _ _ _ _ _ _ _ _ _ _ _ _ _ w1523]
      dyn-events: [_ _ _ _ _ _ _ _ _ _ _ _ _ _ _ w1522] -> w1452
      timeout: _ -> [_ _ _ _ _ _ _ _ _ _ _ _ _ _ _ _]
      tunnel: [_ _ _ _ _ _ _ _ _ _ _ _ _ _ _ w1526] -> w1450
      tunnel: w1454 -> [w1459 w1461 w1466 w1471 w1475 w1479 w1483 w1487 w1493 w1497 w1502 w1506 w1511 w1515 w1520 w1527]
      tunnel: [w1458 _ w1465 w1470 w1472 w1476 w1480 _ w1491 w1494 w1498 w1503 w1507 w1512 w1517 _] -> w1451
      tunnel: [w1457 w1461 w1464 w1469 w1474 w1478 w1482 w1486 w1492 w1495 w1500 w1505 w1508 w1514 w1518 w1527] -> w1449
      event Panel Close? {
        n628 = event-data() -> ()  [unwired: 1 in, 1 out]
        n629 = call-poly "Enqueue Message.vi"("Priority Message? (F)"=TRUE, "Message"="Exit", "Message Queue"=w1459) -> ("error out"=w1458:errorcluster, "dup Message Queue"=w1457:refnum<queue>)  [unwired: 7 in]
        n630 = event-data("Discard?"=TRUE) -> ()  [unwired: 1 in, 1 out]
      }
      event Application Instance Close {
        n631 = event-data() -> ()  [unwired: 1 in, 1 out]
      }
      event "Shutdown": Value Change {
        n632 = event-data() -> ()  [unwired: 1 in, 1 out]
        n633 = call-poly "Enqueue Message.vi"("Priority Message? (F)"=TRUE, "Message"="Exit", "Message Queue"=w1466) -> ("error out"=w1465:errorcluster, "dup Message Queue"=w1464:refnum<queue>)  [unwired: 7 in]
      }
      event "Abort": Value Change {
        n634 = event-data() -> ()  [unwired: 1 in, 1 out]
        n635 = call-poly "Enqueue Message.vi"("Priority Message? (F)"=TRUE, "Message"="Abort", "Message Queue"=w1471) -> ("error out"=w1470:errorcluster, "dup Message Queue"=w1469:refnum<queue>)  [unwired: 7 in]
      }
      event "Select None": Value Change {
        n636 = event-data() -> ()  [unwired: 1 in, 1 out]
        n637 = call-poly "Enqueue Message.vi"("Message"="Select None", "Message Queue"=w1475) -> ("error out"=w1472:errorcluster, "dup Message Queue"=w1474:refnum<queue>)  [unwired: 8 in]
      }
      event "Back": Value Change {
        n638 = event-data() -> ()  [unwired: 1 in, 1 out]
        n639 = call-poly "Enqueue Message.vi"("Message"="Reverse Phase", "Message Queue"=w1479) -> ("error out"=w1476:errorcluster, "dup Message Queue"=w1478:refnum<queue>)  [unwired: 8 in]
      }
      event "Components to build": Value Change {
        n640 = event-data() -> ()  [unwired: 1 in, 1 out]
        n641 = call-poly "Enqueue Message.vi"("Message Data"="Components to build", "Message"="Update Components To Build", "Message Queue"=w1483) -> ("error out"=w1480:errorcluster, "dup Message Queue"=w1482:refnum<queue>)  [unwired: 7 in]
      }
      event "Sync Action": Value Change {
        n642 = event-data() -> ()  [unwired: 1 in, 1 out]
        n643 = call-poly "Enqueue Message.vi"("Message Data"="Sync Action", "Message"="Update Sync Action", "Message Queue"=w1487) -> ("dup Message Queue"=w1486:refnum<queue>)  [unwired: 7 in, 1 out]
      }
      event Value Change {
        n644 = event-data() -> ()  [unwired: 1 in, 1 out]
        n645 = call-poly "Enqueue Message.vi"("Message Data"="Component \\ Export View", "Message"="Update Selection View Type", "Message Queue"=w1493) -> ("error out"=w1491:errorcluster, "dup Message Queue"=w1492:refnum<queue>)  [unwired: 7 in]
      }
      event "Select all": Value Change {
        n646 = event-data() -> ()  [unwired: 1 in, 1 out]
        n647 = call-poly "Enqueue Message.vi"("Message"="Select All", "Message Queue"=w1497) -> ("error out"=w1494:errorcluster, "dup Message Queue"=w1495:refnum<queue>)  [unwired: 8 in]
      }
      event "Build Type": Value Change {
        n648 = event-data() -> ()  [unwired: 1 in, 1 out]
        n649 = call-poly "Enqueue Message.vi"("Message Data"="Build Type", "Message"="Update Build Type", "Message Queue"=w1502) -> ("error out"=w1498:errorcluster, "dup Message Queue"=w1500:refnum<queue>)  [unwired: 7 in]
      }
      event "Next Button": Value Change {
        n650 = event-data() -> ()  [unwired: 1 in, 1 out]
        n651 = call-poly "Enqueue Message.vi"("Message"="Advance Phase", "Message Queue"=w1506) -> ("error out"=w1503:errorcluster, "dup Message Queue"=w1505:refnum<queue>)  [unwired: 8 in]
      }
      event "Successful Builds": Value Change {
        n652 = event-data() -> ()  [unwired: 1 in, 1 out]
        n653 = call-poly "Enqueue Message.vi"("Message Data"="Successful Builds", "Message"="Update Selected Successful Build", "Message Queue"=w1511) -> ("error out"=w1507:errorcluster, "dup Message Queue"=w1508:refnum<queue>)  [unwired: 7 in]
      }
      event "Failed Builds": Value Change {
        n654 = event-data() -> ()  [unwired: 1 in, 1 out]
        n655 = call-poly "Enqueue Message.vi"("Message Data"="Failed Builds", "Message"="Update Selected Failed Build", "Message Queue"=w1515) -> ("error out"=w1512:errorcluster, "dup Message Queue"=w1514:refnum<queue>)  [unwired: 7 in]
      }
      event "Submission Status": Value Change {
        n656 = event-data() -> ()  [unwired: 1 in, 1 out]
        n657 = call-poly "Enqueue Message.vi"("Message Data"="Submission Status", "Message"="Submission Status Val Change", "Message Queue"=w1520) -> ("error out"=w1517:errorcluster, "dup Message Queue"=w1518:refnum<queue>)  [unwired: 7 in]
      }
      event User Event {
        n658 = event-data() -> ("Message"=w1525:string, "Message Data"=w1524:variant)  [unwired: 1 in]
        n659 = case shown="\"Exit\"" w1525 {
          tunnel: [_ TRUE ("Discard?")] -> w1526
          tunnel: w1524 -> [_ _]
          tunnel: w1523 -> [w1528 w1529]
          tunnel: [w1528 w1529] -> w1522
          frame "False", Default {
          }
          frame "Exit" {
          }
        }
      }
    }
    n660 = call "Error Handler - Event Handling Loop.vi"("error in (no error)"=w1451, "Message Queue"=w1449) -> ("dup error in"=w1448:errorcluster)  [unwired: 8 in, 1 out]
  }
  n661 = while {
    tunnel: w10 -> [w1536]
    shift-right: [w1542] -> _
    shift-left: w1 -> [w1543]
    tunnel: w11 -> [w1540]
    tunnel: [w1534] -> w23
    tunnel: w6 -> [w1532]
    tunnel: w5 -> [w1531]
    stop <- w1541 stop-if-true
    # "Appliction Model"
    n662 = call "Dequeue Message.vi"("error in (no error)"=w1540, "Message Queue"=w1536) -> ("error out"=w1539:errorcluster, "Message Data"=w1537:variant, "Message"=w1538:string, "dup Message Queue"=w1535:refnum<queue>)  [unwired: 6 in]
    n663 = case "Message Cases" shown="\"Advance Phase\"" w1538 {
      selector: w1538 -> [_ w1546 w1564 _ _ w1635 w1641 w1647 w1652 _ _ w1679 w1685 w1690]
      tunnel: w1535 -> [_ _ _ w1566 _ w1632 _ _ _ _ w1665 w1683 _ _]
      tunnel: w1539 -> [w1545 w1549 _ w1574 w1611 w1638 _ _ w1654 w1656 w1673 w1680 w1689 _]
      tunnel: [w1545 w1549 w1552 w1574 w1610 w1638 w1639 w1645 w1654 w1655 w1666 w1681 w1689 w1691] -> w1533
      tunnel: w1543 -> [w1544 w1548 w1560 w1570 w1614 w1637 w1643 w1648 w1653 w1660 w1672 w1675 w1688 w1692]
      tunnel: [w1544 w1548 w1559 w1569 w1613 w1637 w1643 w1648 w1653 w1658 w1672 w1675 w1688 w1692] -> w1542
      tunnel: [_ _ _ _ _ _ _ _ _ _ _ TRUE _ _] -> w1541
      tunnel: w1537 -> [_ _ w1561 w1568 _ w1634 w1640 w1646 _ w1661 w1671 _ _ _]
      tunnel: w1532 -> [_ _ _ w1571 w1615 _ _ w1644 w1650 _ _ w1677 w1687 _]
      tunnel: w1531 -> [_ w1547 w1557 w1572 w1616 w1636 w1642 _ w1651 _ _ w1676 w1686 _]
      frame "Initialize" {
        # "Initialize - Send separate messages to initialize the data and the front panel.  Bundle control references."
      }
      frame "Analysis Begin", "Select All" {
        n664 = call-poly "Enqueue Message.vi"("Message"=w1546, "Message Queue"=w1547) -> ()  [unwired: 8 in, 2 out]
      }
      frame "Analysis Complete" {
        n665 = Variant To Data(type=refnum<class "Build Analyzer.lvclass"> refnum ("Build Analyzer"), Variant=w1561) -> (data=w1558:refnum<class "Build Analyzer.lvclass">, error out=w1556:errorcluster)  [unwired: 1 in]
        n666 = Bundle By Name(cluster=w1560, "Build Analyzer"=w1558) -> (w1559:T9)
        n667 = call-poly "Enqueue Message.vi"("error in (no error)"=w1556, "Message"=w1564, "Message Queue"=w1557) -> ("error out"=w1555:errorcluster, "dup Message Queue"=w1563:refnum<queue>)  [unwired: 7 in]
        n668 = call-poly "Enqueue Message.vi"("error in (no error)"=w1555, "Message Data"=w1558, "Message"="Pass Build Analysis", "Message Queue"=w1563) -> ("error out"=w1553:errorcluster, "dup Message Queue"=w1550:refnum<queue>)  [unwired: 6 in]
        n669 = call-poly "Enqueue Message.vi"("error in (no error)"=w1553, "Message"="Populate Components To Build", "Message Queue"=w1550) -> ("error out"=w1552:errorcluster)  [unwired: 7 in, 1 out]
      }
      frame "Advance Phase" {
        n670 = Unbundle By Name(w1570) -> ("Current Phase"=w1573:T8, "Export Build Order"=w1565:refnum<class "Export.lvclass">[])
        n671 = case shown="\"Finished\"" w1573 {
          selector: w1573 -> [_ _ _ _ w1606]
          tunnel: w1572 -> [w1578 w1584 w1594 w1604 w1609]
          tunnel: w1571 -> [w1579 w1581 _ w1605 _]
          tunnel: w1568 -> [_ _ w1593 _ w1607]
          tunnel: [Application_Model_Build_States."Build Pre Check" ("Current Phase") Application_Model_Build_States."Build Status" ("Current Phase") Application_Model_Build_States."Build Results" ("Current Phase") Application_Model_Build_States."Finished" ("Current Phase") w1606] -> w1567
          tunnel: w1566 -> [_ _ w1586 _ _]
          tunnel: w1565 -> [w1575 _ _ _ _]
          frame "Configure Build", Default {
            w1577 = "Pre Build Check" ("Message")
            n672 = call-poly "Enqueue Message.vi"("Message"=w1577, "Message Queue"=w1578) -> ()  [unwired: 8 in, 2 out]
            n673 = call-poly "Enqueue Message.vi"("Message Data"=w1575, "Message"=w1577, "Message Queue"=w1579) -> ()  [unwired: 7 in, 2 out]
          }
          frame "Build Pre Check" {
            w1583 = "Init Build" ("Message")
            n674 = call-poly "Enqueue Message.vi"("Message"=w1583, "Message Queue"=w1584) -> ("error out"=w1580:errorcluster)  [unwired: 8 in, 1 out]
            n675 = call-poly "Enqueue Message.vi"("error in (no error)"=w1580, "Message"=w1583, "Message Queue"=w1581) -> ()  [unwired: 7 in, 2 out]
          }
          frame "Build Status" {
            n676 = call-poly "Enqueue Message.vi"("Message Data"=w1593, "Message"="Build Complete", "Message Queue"=w1594) -> ("dup Message Queue"=w1589:refnum<queue>)  [unwired: 7 in, 1 out]
            n677 = case shown="\"Email On Any Failure\", Default" "Email Behavior" {
              selector: "Email Behavior" -> [_ w1600]
              tunnel: w1589 -> [w1597 w1601]
              tunnel: [w1597 w1599] -> _
              tunnel: "Send Email" ("Message") -> [_ w1598]
              frame "Do Not Email" {
              }
              frame "Email On Any Failure", Default {
                n678 = call-poly "Enqueue Message.vi"("Message Data"=w1600, "Message"=w1598, "Message Queue"=w1601) -> ("dup Message Queue"=w1599:refnum<queue>)  [unwired: 7 in, 1 out]
              }
            }
            n679 = case shown="\"Auto Submit All Built Exports\"" "Auto Submit Behavior" {
              tunnel: w1586 -> [w1596 _]
              tunnel: "Advance Phase" ("Message") -> [w1595 _]
              frame "Auto Submit All Built Exports" {
                n680 = call-poly "Enqueue Message.vi"("Message"=w1595, "Message Queue"=w1596) -> ()  [unwired: 8 in, 2 out]
              }
              frame "No Auto Submit", Default {
              }
            }
          }
          frame "Build Results" {
            w1603 = "Commit" ("Message")
            n681 = call-poly "Enqueue Message.vi"("Message"=w1603, "Message Queue"=w1604) -> ()  [unwired: 8 in, 2 out]
            n682 = call-poly "Enqueue Message.vi"("Message"=w1603, "Message Queue"=w1605) -> ()  [unwired: 8 in, 2 out]
          }
          frame "Finished" {
            n683 = call-poly "Enqueue Message.vi"("Message Data"=w1607, "Message"="Finished", "Message Queue"=w1609) -> ()  [unwired: 7 in, 2 out]
          }
        }
        n684 = Bundle By Name(cluster=w1570, "Current Phase"=w1567) -> (w1569:T9)
      }
      frame "Reverse Phase" {
        n685 = Unbundle By Name(w1614) -> ("Current Phase"=w1617:T8)
        n686 = case shown="\"Build Results\"" w1617 {
          selector: w1617 -> [w1619 w1621 _ _]
          tunnel: w1616 -> [_ _ w1626 w1631]
          tunnel: w1615 -> [_ _ w1625 _]
          tunnel: [w1619 w1621 Application_Model_Build_States."Configure Build" ("Current Phase") Application_Model_Build_States."Configure Build" ("Current Phase")] -> w1612
          tunnel: w1611 -> [w1618 w1620 w1622 w1628]
          tunnel: [w1618 w1620 w1622 w1628] -> w1610
          frame "Configure Build", Default {
          }
          frame "Build Status" {
          }
          frame "Build Results" {
            n687 = call-poly "Enqueue Message.vi"("Message"="Reconfigure Build", "Message Queue"=w1626) -> ()  [unwired: 8 in, 2 out]
            n688 = call-poly "Enqueue Message.vi"("Message"="Clean Exports", "Message Queue"=w1625) -> ()  [unwired: 8 in, 2 out]
          }
          frame "Finished" {
            n689 = call-poly "Enqueue Message.vi"("Message"="Restart", "Message Queue"=w1631) -> ()  [unwired: 8 in, 2 out]
          }
        }
        n690 = Bundle By Name(cluster=w1614, "Current Phase"=w1612) -> (w1613:T9)
      }
      frame "Pre Build Commit Readiness Failure" {
        n691 = call-poly "Enqueue Message.vi"("Message"="Exit", "Message Queue"=w1632) -> ()  [unwired: 8 in, 2 out]
        n692 = call-poly "Enqueue Message.vi"("Message Data"=w1634, "Message"=w1635, "Message Queue"=w1636) -> ()  [unwired: 7 in, 2 out]
      }
      frame "Commit Complete", "Commit Readiness Failure", "Exports Cleaned", "Final Build Status", "Submission Status Val Change", "Update Build Marker", "Update Build Type", "Update Components To Build", "Update Email Behavior", "Update Selected Failed Build", "Update Selected Successful Build", "Update Selection View Type" {
        n693 = call-poly "Enqueue Message.vi"("Message Data"=w1640, "Message"=w1641, "Message Queue"=w1642) -> ("error out"=w1639:errorcluster)  [unwired: 7 in, 1 out]
      }
      frame "Update Sync Action" {
        n694 = call-poly "Enqueue Message.vi"("Message Data"=w1646, "Message"=w1647, "Message Queue"=w1644) -> ("error out"=w1645:errorcluster)  [unwired: 7 in, 1 out]
      }
      frame "Select None" {
        n695 = call-poly "Enqueue Message.vi"("Message"=w1652, "Message Queue"=w1651) -> ()  [unwired: 8 in, 2 out]
        n696 = call-poly "Enqueue Message.vi"("Message"="Flush Ordered Exports", "Message Queue"=w1650) -> ()  [unwired: 8 in, 2 out]
      }
      frame "New Ordered Exports Available" {
        n697 = Unbundle By Name(w1660) -> ("Export Build Order"=w1659:refnum<class "Export.lvclass">[])
        n698 = Variant To Data(error in=w1656, type=w1659, Variant=w1661) -> (data=w1657:refnum<class "Export.lvclass">[], error out=w1655:errorcluster)
        n699 = Bundle By Name(cluster=w1660, "Export Build Order"=w1657) -> (w1658:T9)
      }
      frame "Error" {
        # "Error - Check the error message data and respond accordingly. This message is sent by the \"Error Handler\" VIs at the end of each loop in this application."
        n700 = Variant To Data(error in=w1673, type=errorcluster {"status"=FALSE, "code"=0, "source"=""} ("error constant"), Variant=w1671) -> (data=w1669:errorcluster, error out=w1668:errorcluster)
        n701 = call <vilib>:"Simple Error Handler.vi"("error source (\" \")"="Application Model" ("error source (\" \")"), "error in (no error)"=w1669) -> ()  [unwired: 3 in, 5 out]
        n702 = call-poly "Enqueue Message.vi"("Priority Message? (F)"=TRUE, "Message"="Exit", "Message Queue"=w1665) -> ("error out"=w1667:errorcluster)  [unwired: 7 in, 1 out]
        n703 = Merge Errors(w1667, w1668) -> (w1666:errorcluster)
      }
      frame "Exit" {
        # "Exit - Exit the application."
        n704 = Unbundle By Name(w1675) -> ("Dynamic Event"=w1674:refnum<user-event>)
        n705 = Generate User Event(user event=w1674, event data cluster=T10 {"Message"="Exit", "Message Data"=variant} ("event data")) -> ()  [unwired: 2 in, 2 out]
        n706 = call-poly "Enqueue Message.vi"("Message"=w1679, "Message Queue"=w1677) -> ()  [unwired: 8 in, 2 out]
        n707 = call-poly "Enqueue Message.vi"("Message"=w1679, "Message Queue"=w1676) -> ()  [unwired: 8 in, 2 out]
        n708 = Release Queue(queue=w1683, error in (no error)=w1680) -> (error out=w1681:errorcluster)  [unwired: 1 in, 2 out]
      }
      frame "Abort" {
        n709 = call-poly "Enqueue Message.vi"("Message"=w1685, "Message Queue"=w1686) -> ()  [unwired: 8 in, 2 out]
        n710 = call-poly "Enqueue Message.vi"("Priority Message? (F)"=TRUE, "Message"=w1685, "Message Queue"=w1687) -> ()  [unwired: 7 in, 2 out]
      }
      frame Default {
        # "'Default' case only runs if there is a message that isn't defined in any of the other cases.  Output a programming error."
        n711 = xnode "Error Ring"("parameter 0"=w1690) -> ("error out"=w1691:errorcluster)
      }
    }
    n712 = call "Error Handler - Message Handling Loop.vi"("error in (no error)"=w1533, "Message Queue"=w1535) -> ("dup error in"=w1534:errorcluster)  [unwired: 8 in, 1 out]
  }
  n713 = Unregister For Events(event registration refnum=w9, error in=w8) -> (error out=w22:errorcluster)
  n714 = Merge Errors(w22, w23, w18, w17) -> (w16:errorcluster)
  n715 = Destroy User Event(user event=w13, error in=w16) -> ()  [unwired: 1 out]
